vi "DB UI - Admin Equipment.vi"() -> ()   [LabVIEW 2013]
uses:
  Controls/Combo Box.ctl
  <vilib>/Utility/miscctls.llb/LVRowAndColumnUnsignedTypeDef.ctl
  <vilib>/Utility/miscctls.llb/LVRowAndColumnTypeDef.ctl
  <vilib>/Utility/miscctls.llb/LVPointTypeDef.ctl
  Controls/DB - [Admin].[Equipment] v20140922_1553.ctl
  Controls/Global SRTRS.vi
  <vilib>/addons/database/Connection.llb/DB Tools Open Connec (String).vi
  <vilib>/addons/database/Connection.llb/Conn Execute.vi
  <vilib>/addons/database/Recordset.llb/Rec Destroy - Connection.vi
  <vilib>/addons/database/Recordset.llb/Rec Fetch Recordset Data (R).vi
  <vilib>/addons/database/_DB Variant To Data/Database Variant To Data.xnode
  <vilib>/addons/database/NI_Database_API.lvlib
panel:
  in  "Search Equipment ID":T1
  in  "Tab Control":enum32{"Debug"}(tab)
  out "MHandler":errorcluster
  in  "Stop Button":bool
  out "Statemachine":errorcluster
  in  "# of Columns":i32=8
  out "Primary Keys":string[](array[string])=["OrderNo"]
  out "Foreign Keys":string[](array[string])=["OrderNo"]
  in  "Next Button":bool
  in  "Previous Button":bool
  out "1st Primary KEY":string
  in  "Last Button":bool
  in  "First Button":bool
  out "datetime string":string
  out "Changed":bool
  out "SQL Query":string
  in  "Include Inactive":bool=TRUE
  out "Extra Event From \"Select Foreign Key\"":bool
  out "IDENTITY COLUMN":string
  out "Close":errorcluster
  out "New Record in UI not in DB":bool
  out "Property Node":errorcluster
  out "DB":errorcluster
  in  "DB.Schema.Table":string="SRTRS.Admin.Equipment"
  in  "[PlantId]":string="4070"
  in  "DB.Schema.Table 2":string="SRTRS.Config.EquipmentType"
  in  "DB.Schema.Table 3":string="SRTRS.Config.System"
  out "Col Hdrs[] DB Data Type":string[](array[string])
  in  "# of Rows":u32=8
  out "Col Hdrs[] DB Precision":string[](array[string])
  out "All Mandatory Fields Filled":bool
  in  "------------------------------------        User Details Header EVENTS     ------------------------------------":string caption="------------------------------------        Setup Tab     ------------------------------------"
  in  "------------------------------------------        Unused EVENTS     ----------------------------------------":string caption="------------------------------------        Setup Tab     ------------------------------------"
  out "Connection Information":T2={"Connection "="SQL Server 32bit HPEnvy", "Username"="admin", "Password"="admin123"}
  out "MCListBox":u32
  out "NewVal":i32
  out "User Details":u32
  out "Controls (Caption) that are blank (Unicode)":string[](array[string])
  in  "Save Enabled depends on \nFilled Mandatory Fields":bool
  in  "CellBG New Cells":u32(colorbox)=16777225
  in  "CellBG Unused Cells":u32(colorbox)=16777238
  in  "CellBG ColHdrs":u32(colorbox)=11776947
  in  "Ascending":bool
  in  "List [CaptionOnly]":string caption="List"
  in  "Cal. History":bool caption="Setup Save"
  in  "Search System ID":T1
  in  "Save":bool caption="Setup Save"
  in  "New":bool caption="Setup Save"
  in  "Equipment Details Cluster":T3={"Equipment ID"="", "Equipment Name"="", "Plant ID"="", "Equipment Type"="", "System"="", "Manufacturer"="", "Model Number"="", "Serial Number"="", "Last Calibration"=timestamp(0 s since 1904-01-01), "Next Calibration"=timestamp(0 s since 1904-01-01), "Calibration Period"="", "Notice Period"="", "Registration Date"=timestamp(0 s since 1904-01-01), "Remarks"="", "Out For Calibration"=FALSE, "Required Calibration"=TRUE, "Inactive"=FALSE, "Equipment Type Name"="", "System Name"="", "Days1 [CaptionOnly]"="", "Days2 [CaptionOnly]"=""} caption="Record" {"Registration Date" format="%<%Y/%m/%d>T"; "Last Calibration" format="%<%Y/%m/%d>T"; "Next Calibration" format="%<%Y/%m/%d>T"}
  in  "Current Record":i32 caption="No."
  out "Record Count":i32
  in  "Multicolumn Listbox":i32(listbox)=3
  # "/"
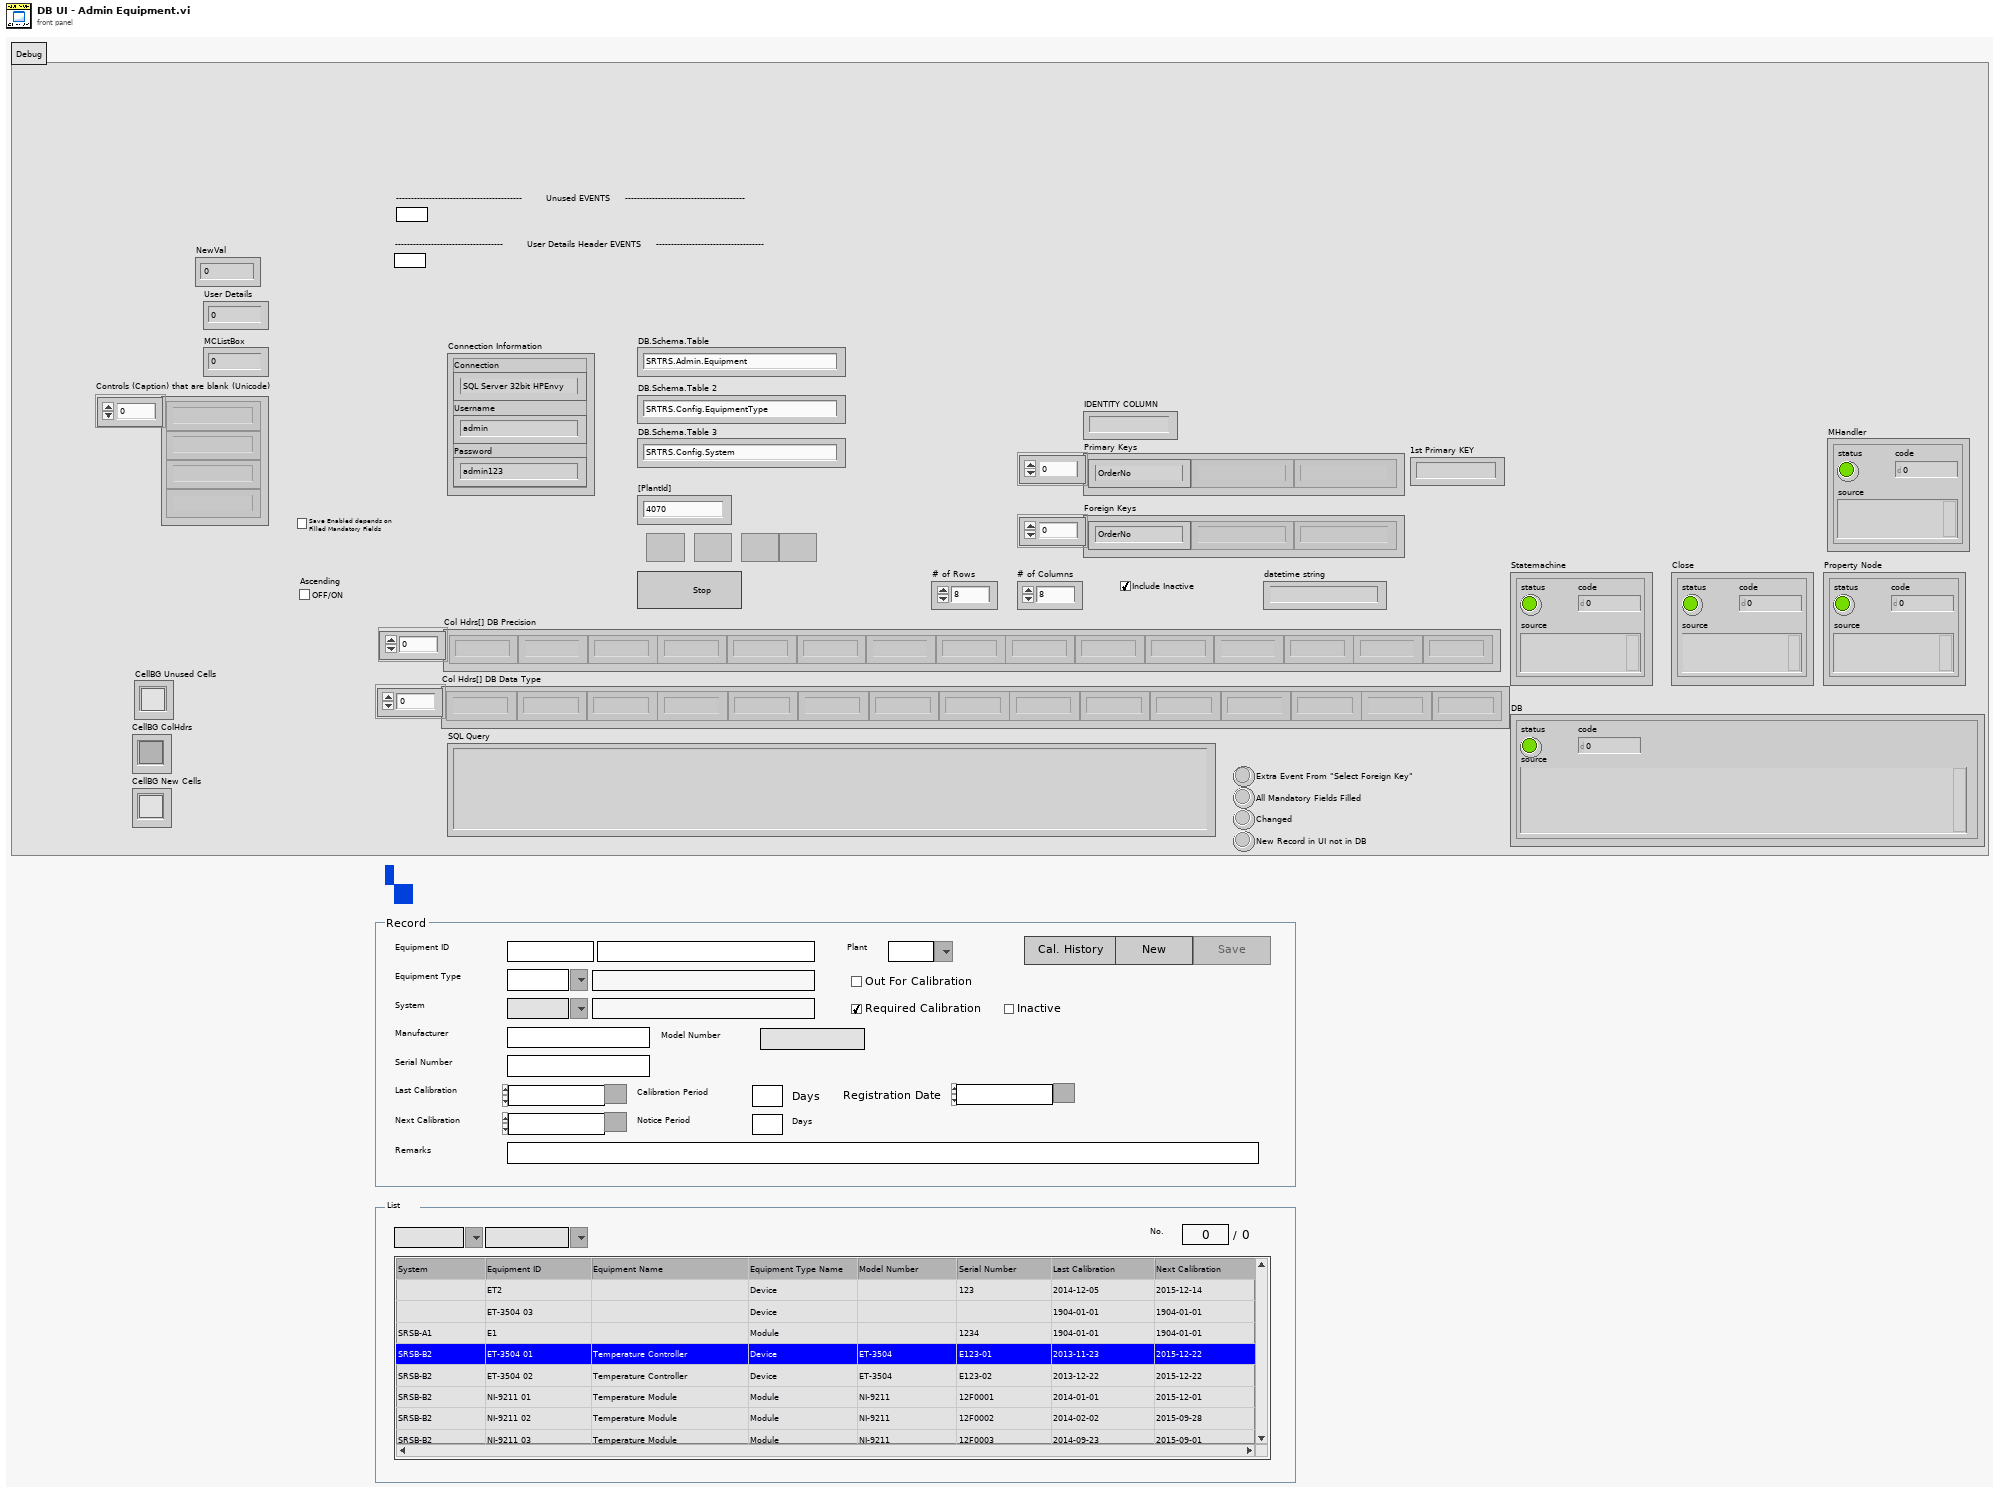
[diagram p1: front panel]
types:
  T1 = typedef "Combo Box.ctl" = string
  T2 = cluster{"Connection ":string, "Username":string, "Password":string}
  T3 = cluster{"Equipment ID":string, "Equipment Name":string, "Plant ID":T1, "Equipment Type":T1, "System":T1, "Manufacturer":string, "Model Number":string, "Serial Number":string, "Last Calibration":timestamp, "Next Calibration":timestamp, "Calibration Period":string, "Notice Period":string, "Registration Date":timestamp, "Remarks":string, "Out For Calibration":bool, "Required Calibration":bool, "Inactive":bool, "Equipment Type Name":string, "System Name":string, "Days1 [CaptionOnly]":string, "Days2 [CaptionOnly]":string}
  T4 = typedef "LVPointTypeDef.ctl" = cluster{"Horizontal":i16, "Vertical":i16}
  T5 = typedef "LVRowAndColumnUnsignedTypeDef.ctl" = cluster{"Row":u32, "Column":u32}
  T6 = enum8{"Enabled", "Disabled", "Disabled and Grayed Out"}
  T7 = typedef "DB - [Admin].[Equipment] v20140922_1553.ctl" = enum16{"a.[PlantId]", "a.[EquipmentId]", "a.[Description]", "a.[EquipmentTypeId]", "c.[ShortDescription]", "a.[SystemId]", "s.[Description]", "a.[Manufacturer]", "a.[Model]", "a.[SerialNo]", "a.[RegistrationDate]", "a.[IsCalibRequired]", "a.[IsCalibOut]", "a.[CalibrationPeriod]", "a.[NoticePeriod]", "a.[LastCalibDate]", "a.[NextCalibDate]", "a.[Remarks]", "a.[Inactive]"}
  T8 = typedef "LVRowAndColumnTypeDef.ctl" = cluster{"Row":i32, "Column":i32}
  T9 = typedef "Connection Information Cluster.ctl" = cluster{"Connection ":string, "Username":string, "Password":string}
  T10 = typedef "NI_Database_API.lvlib/Conn ObjectReference.ctl" = refnum<k1>
  T11 = typedef "DB - DB.Schema.Table.ctl" = cluster{"DB":string, "Schema":string, "Table":string}
  T12 = typedef "NI_Database_API.lvlib/Rec ObjectReference.ctl" = refnum<k1>
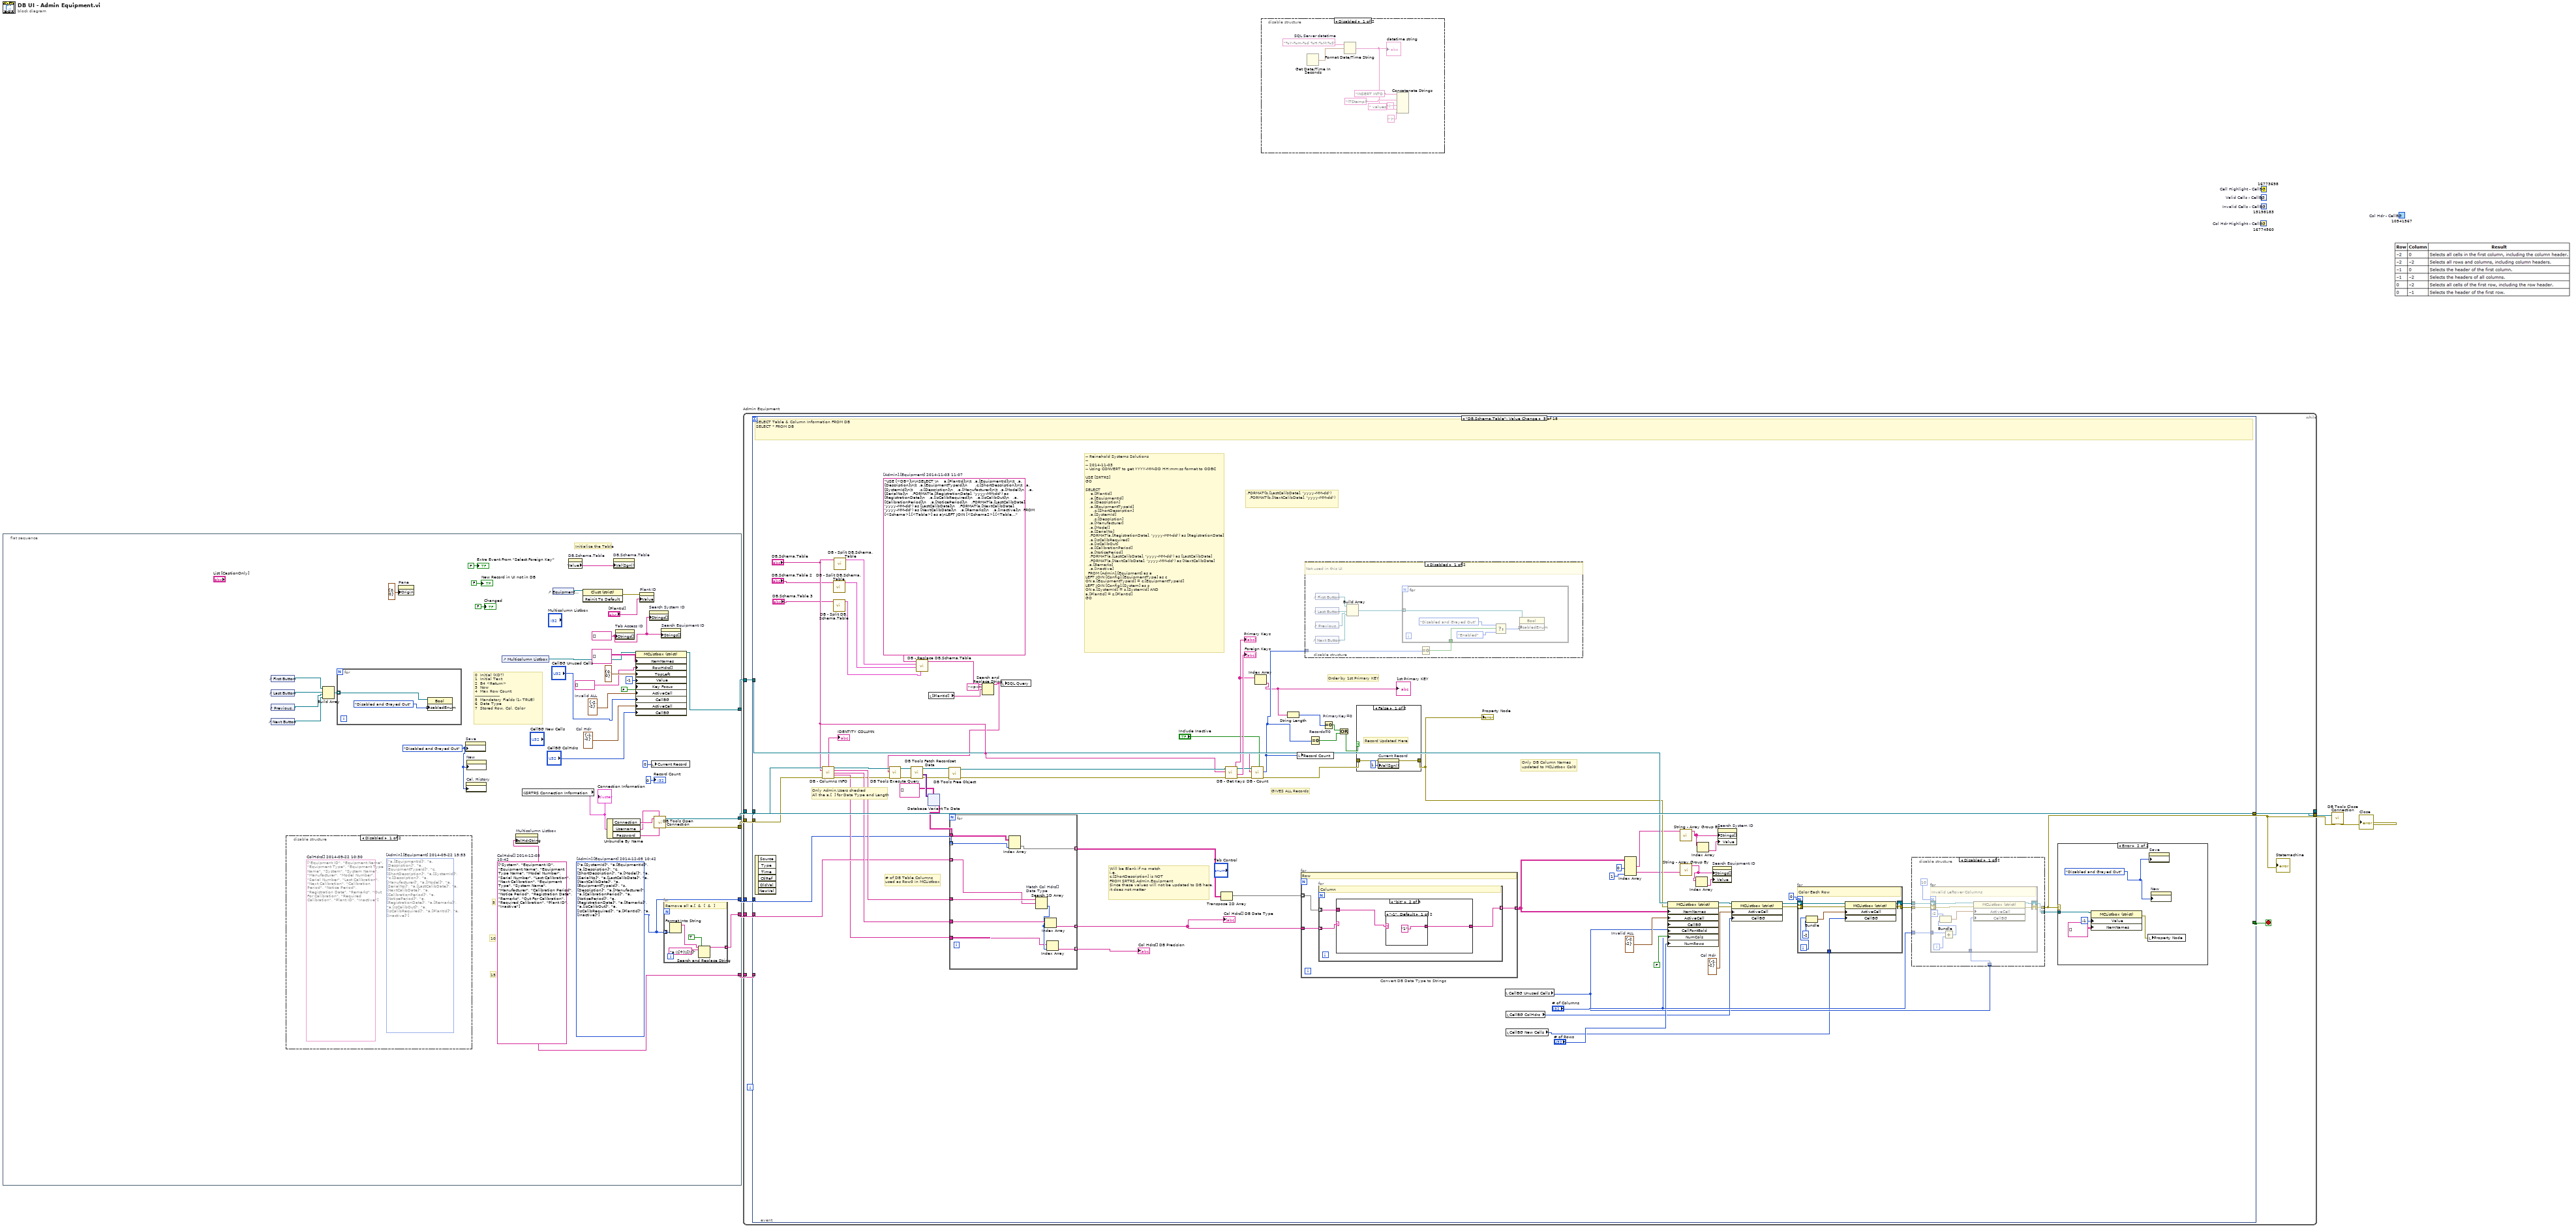
[diagram p0: block diagram]
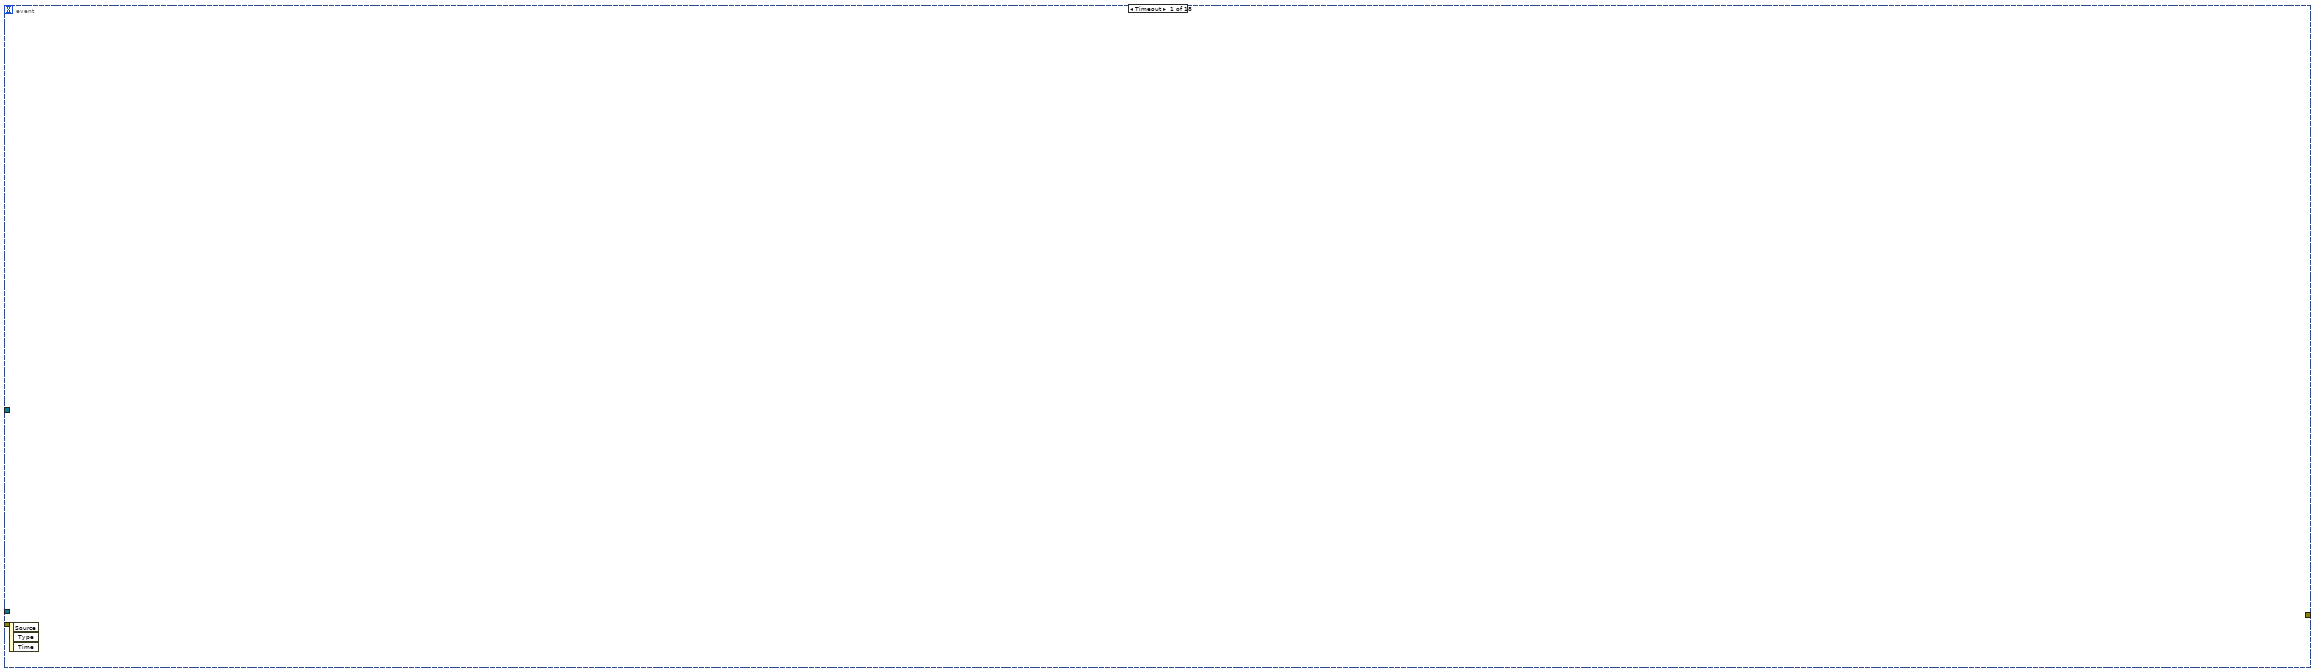
[diagram p4: hidden frame]
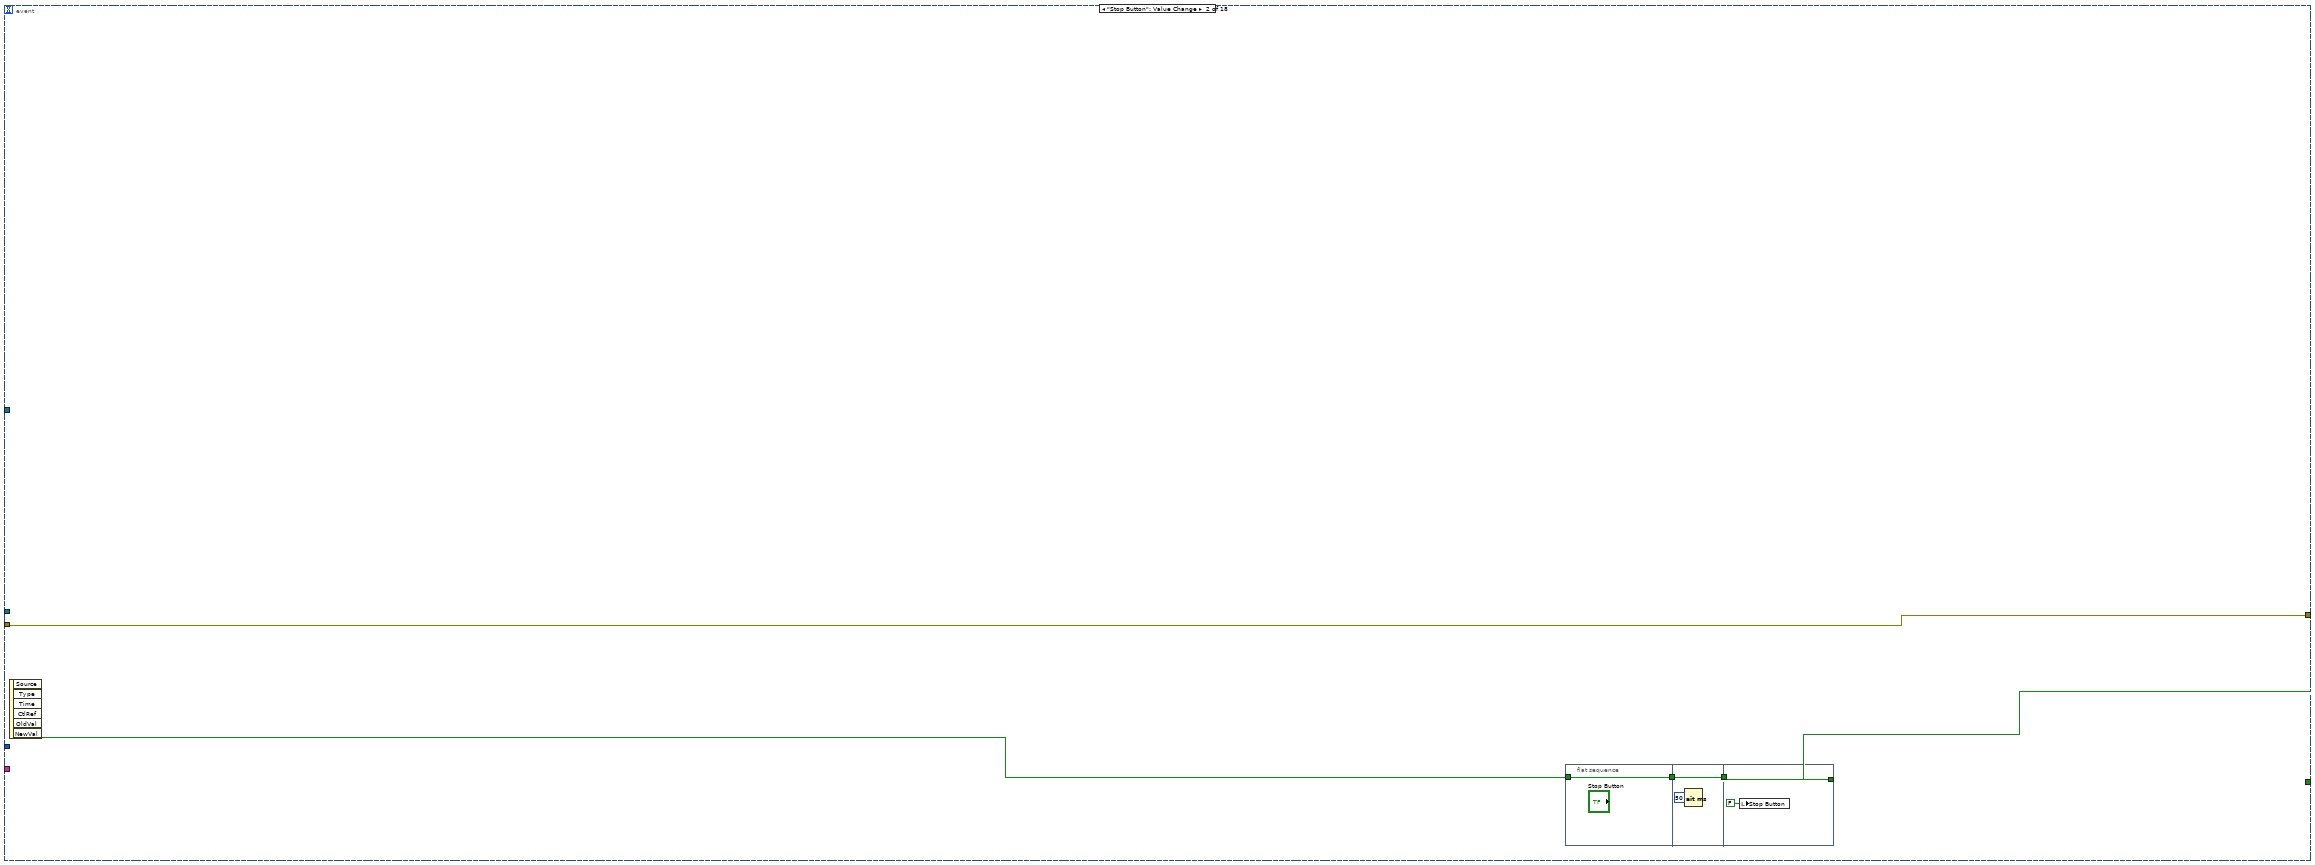
[diagram p5: hidden frame]
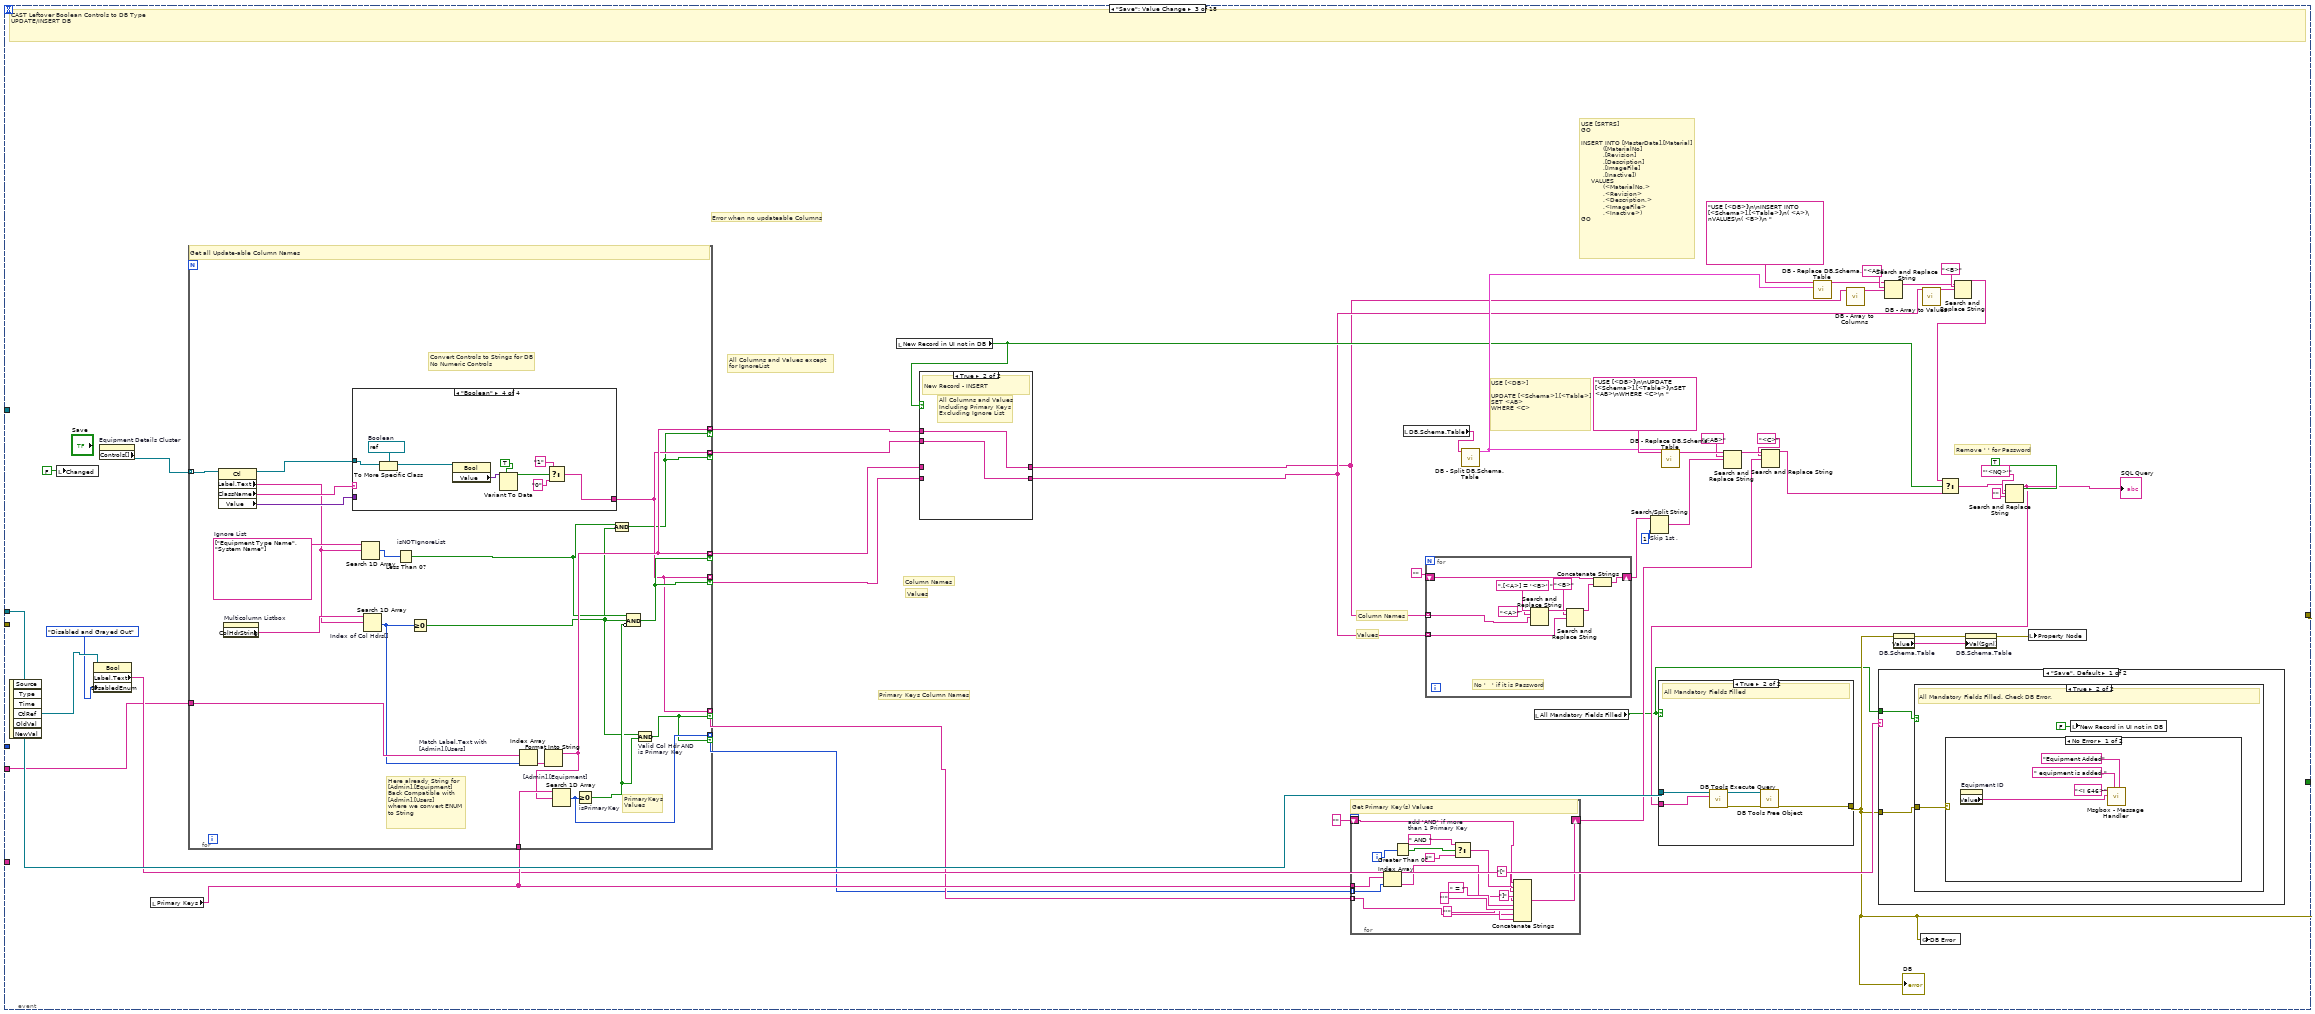
[diagram p6: hidden frame]
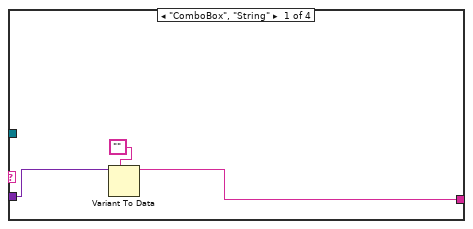
[diagram p8: hidden frame]
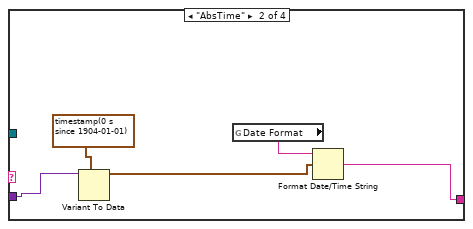
[diagram p9: hidden frame]
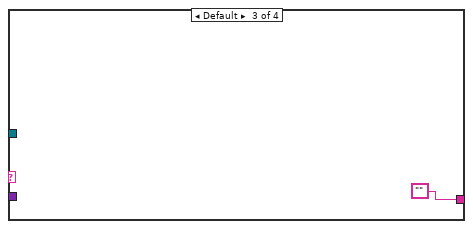
[diagram p10: hidden frame]
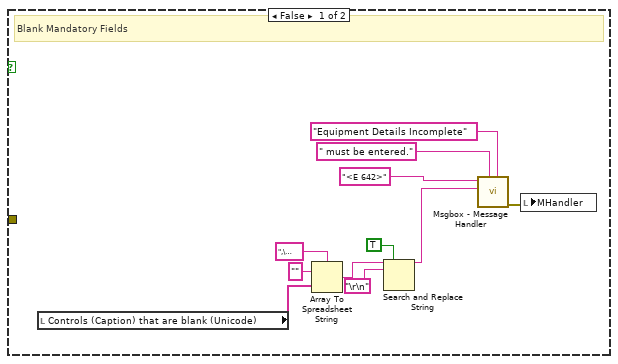
[diagram p12: hidden frame]
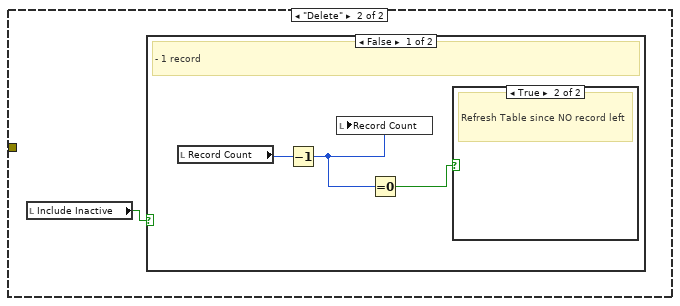
[diagram p14: hidden frame]
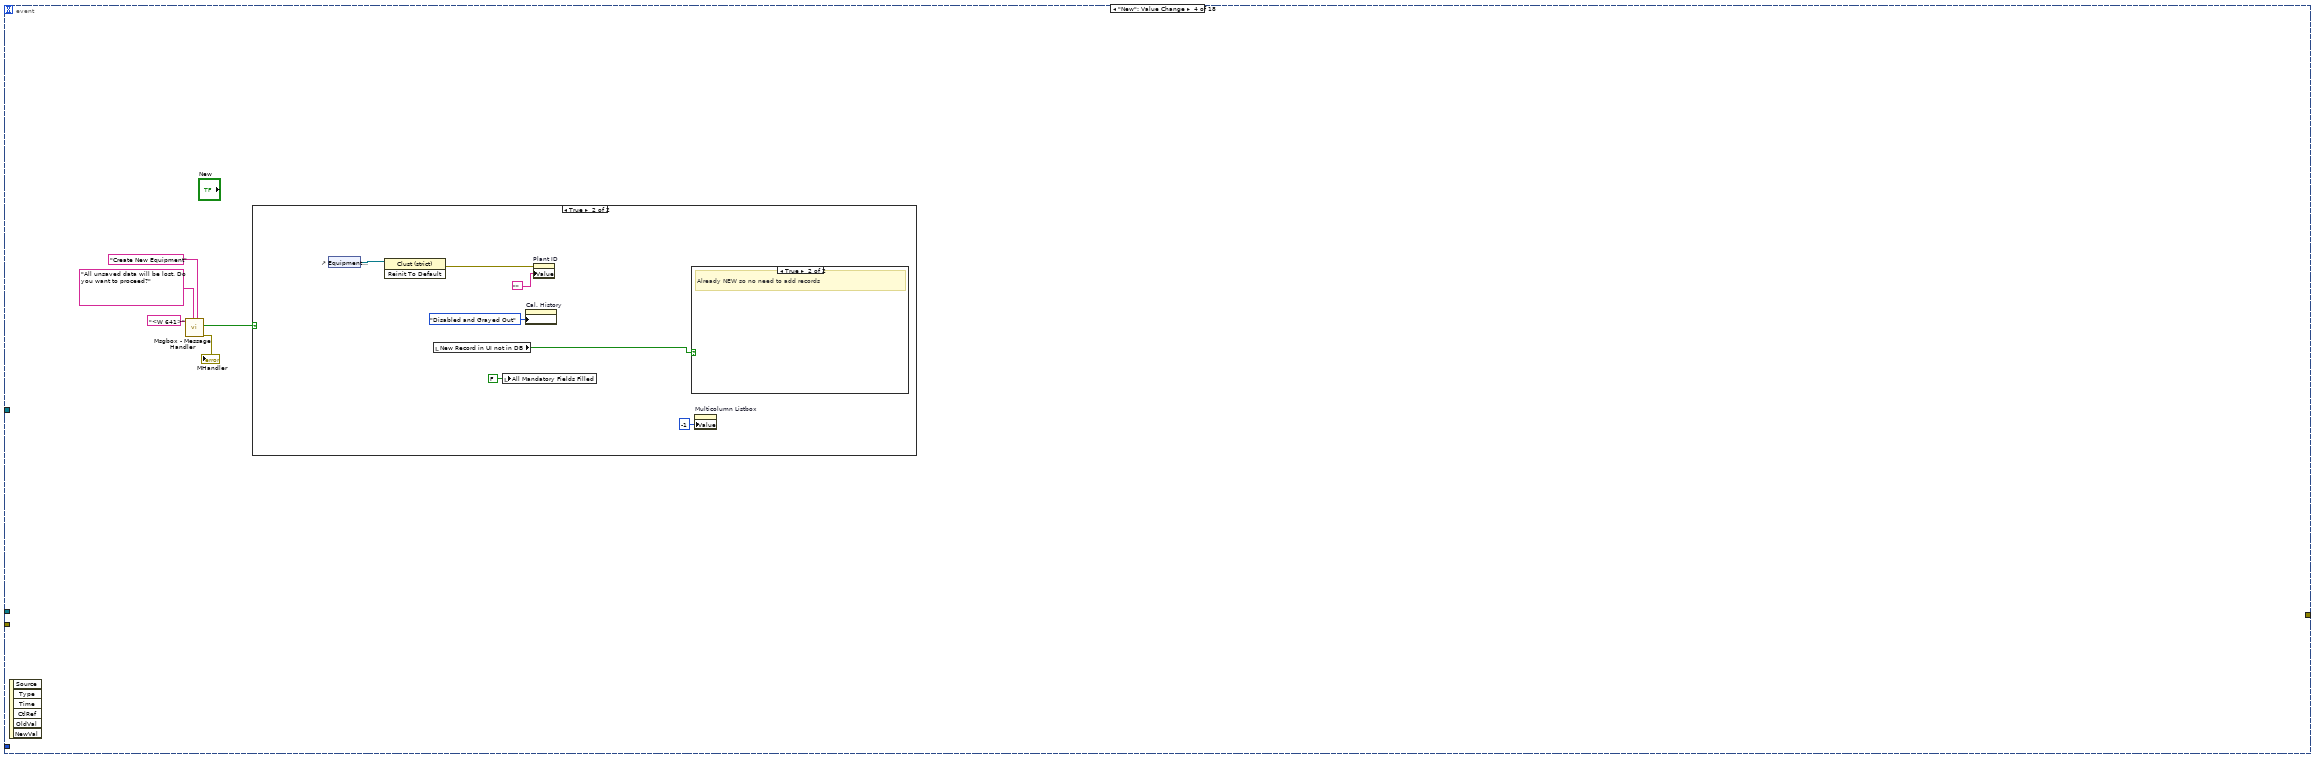
[diagram p17: hidden frame]
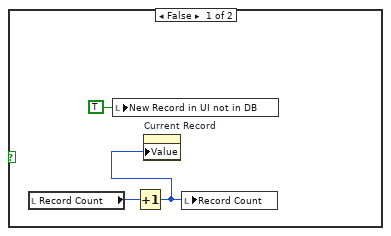
[diagram p19: hidden frame]
diagram:
  (unwired) u32 10541567  # Col Hdr - CellBG
  (unwired) u32 16777226  # Valid Cells - CellBG
  (unwired) u32 15198183  # Invalid Cells - CellBG
  (unwired) u32 16774560  # Col Hdr Highlight - CellBG
  (unwired) u32 16773698  # Cell Highlight - CellBG
  n1 = flat-sequence {
    tunnel: [w43] -> w9
    tunnel: [w23] -> w6
    tunnel: [w41] -> w5
    tunnel: [w16] -> w3
    tunnel: [w19] -> w2
    tunnel: [w15] -> w1
    frame #0 {
      w15 = T7[] [enum."a.[SystemId]", enum."a.[EquipmentId]", enum."a.[Description]", enum."c.[ShortDescription]", enum."a.[Model]", enum."a.[SerialNo]", enum."a.[LastCalibDate]", enum."a.[NextCalibDate]", enum."a.[EquipmentTypeId]", enum."s.[Description]", enum."a.[Manufacturer]", enum."a.[CalibrationPeriod]", enum."a.[NoticePeriod]", enum."a.[RegistrationDate]", enum."a.[Remarks]", enum."a.[IsCalibOut]", enum."a.[IsCalibRequired]", enum."a.[PlantId]", enum."a.[Inactive]"] items=["a.[PlantId]", "a.[EquipmentId]", "a.[Description]", "a.[EquipmentTypeId]", "c.[ShortDescription]", "a.[SystemId]", "s.[Description]", "a.[Manufacturer]", "a.[Model]", "a.[SerialNo]", "a.[RegistrationDate]", "a.[IsCalibRequired]", "a.[IsCalibOut]", "a.[CalibrationPeriod]", "a.[NoticePeriod]", "a.[LastCalibDate]", "a.[NextCalibDate]", "a.[Remarks]", "a.[Inactive]"]  # [Admin].[Equipment] 2014-12-05 10:42
      w10 = string[] [] ("Strings []")
      w19 = string[] ["System", "Equipment ID", "Equipment Name", "Equipment Type Name", "Model Number", "Serial Number", "Last Calibration", "Next Calibration", "Equipment Type", "System Name", "Manufacturer", "Calibration Period", "Notice Period", "Registration Date", "Remarks", "Out For Calibration", "Required Calibration", "Plant ID", "Inactive"]  # ColHdrs[] 2014-12-05 10:42
      w24 = T8 {"Row"=-1, "Column"=-2}  # Col Hdr
      w25 = T8 {"Row"=-2, "Column"=-2}  # Invalid ALL
      w13 = T6."Disabled and Grayed Out" ("Disabled")
      # "15"
      # "10"
      # "5"
      # "Initialize the Table"
      # "0  Initial (KD?)\n1  Initial Text\n2  B4 <Return>\n3  Now\n4  Max Row Count\n-------------------\n5  Mandatory Fields (1- TRUE)\n6  Data Type\n7  Stored Row, Col, Color"
      n2 = control-ref of="First Button"() -> (w37:refnum<vi>)
      n3 = control-ref of="Last Button"() -> (w36:refnum<vi>)
      n4 = control-ref of="Previous Button"() -> (w35:refnum<vi>)
      n5 = control-ref of="Next Button"() -> (w34:refnum<vi>)
      n6 = disable-structure shown="Disabled" {
        frame Disabled {
          (unwired) T7[] [enum."a.[EquipmentId]", enum."a.[Description]", enum."a.[EquipmentTypeId]", enum."c.[ShortDescription]", enum."a.[SystemId]", enum."s.[Description]", enum."a.[Manufacturer]", enum."a.[Model]", enum."a.[SerialNo]", enum."a.[LastCalibDate]", enum."a.[NextCalibDate]", enum."a.[CalibrationPeriod]", enum."a.[NoticePeriod]", enum."a.[RegistrationDate]", enum."a.[Remarks]", enum."a.[IsCalibOut]", enum."a.[IsCalibRequired]", enum."a.[PlantId]", enum."a.[Inactive]"] items=["a.[PlantId]", "a.[EquipmentId]", "a.[Description]", "a.[EquipmentTypeId]", "c.[ShortDescription]", "a.[SystemId]", "s.[Description]", "a.[Manufacturer]", "a.[Model]", "a.[SerialNo]", "a.[RegistrationDate]", "a.[IsCalibRequired]", "a.[IsCalibOut]", "a.[CalibrationPeriod]", "a.[NoticePeriod]", "a.[LastCalibDate]", "a.[NextCalibDate]", "a.[Remarks]", "a.[Inactive]"]  # [Admin].[Equipment] 2014-09-22 15:53
          (unwired) string[] ["Equipment ID", "Equipment Name", "Equipment Type", "Equipment Type Name", "System", "System Name", "Manufacturer", "Model Number", "Serial Number", "Last Calibration", "Next Calibration", "Calibration Period", "Notice Period", "Registration Date", "Remarks", "Out For Calibration", "Required Calibration", "Plant ID", "Inactive"]  # ColHdrs[] 2014-09-22 10:30
        }
        frame Enabled {
        }
      }
      n7 = Build Array(w37, w36, w35, w34) -> (w38:refnum<vi>[])
      n8 = for {
        tunnel: w38 -> [w53] mode=indexing
        n9 = property class="Bool"(reference=w53, "DisabledEnum"=T6."Disabled and Grayed Out" ("Disabled")) -> ()  [unwired: 1 in, 2 out]
      }
      n10 = property on="Pane" class="Pane"("Origin"=T4 {"Horizontal"=0, "Vertical"=0}) -> ()  [unwired: 2 in, 2 out]
      n11 = property on="Save" class="Bool"("DisabledEnum"=w13) -> ()  [unwired: 2 in, 2 out]
      n12 = property on="Cal. History" class="Bool"("DisabledEnum"=w13) -> ()  [unwired: 2 in, 2 out]
      n13 = property on="New" class="Bool"("DisabledEnum"=w13) -> ()  [unwired: 2 in, 2 out]
      n14 = control-ref of="Multicolumn Listbox"() -> (w22:refnum<vi>)
      n15 = property on="Multicolumn Listbox" class="MCListbox (strict)"("ColHdrString"=w19) -> ()  [unwired: 2 in, 2 out]
      n16 = global read "Global SRTRS.vi" "SRTRS Connection Information"() -> (w14:T9)
      "Connection Information" <- w14
      n17 = control-ref of="Equipment Details Cluster"() -> (w21:refnum<vi>)
      n18 = property on="DB.Schema.Table" class="Str"() -> ("Value"=w31:string)  [unwired: 2 in, 2 out]
      n19 = invoke class="Clust (strict)" method="Reinit To Default"(reference=w21) -> (error out=w20:errorcluster)  [unwired: 2 in, 2 out]
      n20 = Unbundle By Name(w14) -> ("Connection"=w46:string, "Username"=w45:string, "Password"=w44:string)
      n21 = property on="DB.Schema.Table" class="Str"("Val(Sgnl)"=w31) -> ()  [unwired: 2 in, 2 out]
      n22 = property on="Tab Access ID" class="CmbBox (strict)"("Strings[]"=w10) -> ()  [unwired: 2 in, 2 out]
      n23 = property on="Property Node" class="MCListbox (strict)"(reference=w22, "ItemNames"=string[][] [] ("Item Names"), "RowHdrs[]"=string[] [] ("Item Names"), "TopLeft"=T5 {"Row"=0, "Column"=0} ("Top Left Visible Cell"), "Value"=-1, "Key Focus"=FALSE, "ActiveCell"=w25, "CellBG"="CellBG Unused Cells", "ActiveCell"=w24, "CellBG"="CellBG ColHdrs") -> (reference out=w23:refnum<vi>)  [unwired: 1 in, 1 out]
      n24 = property on="Plant ID" class="CmbBox (strict)"(error in=w20, "Value"="[PlantId]") -> ()  [unwired: 1 in, 2 out]
      n25 = property on="Search System ID" class="CmbBox (strict)"("Strings[]"=w10) -> ()  [unwired: 2 in, 2 out]
      n26 = local write "Current Record"(0 ("Current Record")) -> ()
      n27 = call-poly <vilib>:"DB Tools Open Connection.vi"("password"=w44, "userID"=w45, "connection information"=w46) -> ("error out"=w41:errorcluster, "connection reference"=w43:T10)  [unwired: 5 in]
      n28 = property on="Search Equipment ID" class="CmbBox (strict)"("Strings[]"=w10) -> ()  [unwired: 2 in, 2 out]
      n29 = for {
        tunnel: w15 -> [w51] mode=indexing
        tunnel: [w47] -> w16 mode=indexing
        # "Remove all a.[  &  [  &  ]"
        n30 = Format Into String(w51) -> (resulting string=w48:string)  [unwired: 3 in, 1 out]
        n31 = Search and Replace String(replace all?=TRUE ("replace all? (F)"), input string=w48, search string="a.\\[+|\\[|\\]") -> (result string=w47:string)  [unwired: 5 in, 3 out]
      }
      "Extra Event From \"Select Foreign Key\"" <- FALSE ("Extra Event From \"Select Foreign Key Value Changed\"")
      "Record Count" <- 0 ("Record Count")
      "New Record in UI not in DB" <- FALSE ("New Record in UI not in DB")
      "Changed" <- FALSE ("Changed")
    }
  }
  n32 = while "Admin Equipment" {
    tunnel: w9 -> [w58]
    tunnel: [w58] -> w8
    tunnel: [w57] -> w7
    tunnel: w5 -> [w60]
    tunnel: w6 -> [w59]
    tunnel: w3 -> [w56]
    tunnel: w2 -> [w55]
    tunnel: w1 -> [w54]
    stop <- w61 stop-if-true
    n33 = event shown="[4] \"DB.Schema.Table\": Value Change" {
      selector: _ -> [_ _ _ _ _ _ _ _ _ _ _ _ _ _ _ _ _ _]
      dyn-events: _ -> [_ _ _ _ _ _ _ _ _ _ _ _ _ _ _ _ _ _]
      timeout: _ -> [_ _ _ _ _ _ _ _ _ _ _ _ _ _ _ _ _ _]
      tunnel: [_ w64 _ _ _ _ _ _ _ _ _ _ _ _ _ _ _ _] -> w61
      tunnel: w58 -> [_ _ w120 _ w293 _ _ _ _ _ _ w564 w630 _ _ _ _ w881]
      tunnel: [_ w66 w73 _ w280 _ _ _ w467 _ _ w545 _ _ _ _ _ _] -> w57
      tunnel: w60 -> [_ w66 _ _ w292 _ _ _ w468 _ _ _ _ _ _ _ _ w880]
      tunnel: w59 -> [_ _ _ _ w301 _ w446 _ w466 _ _ _ _ w720 _ w779 _ _]
      tunnel: w56 -> [_ _ w91 _ w272 _ _ _ _ _ _ w553 w650 _ _ _ _ _]
      tunnel: w55 -> [_ _ _ _ _ _ _ _ _ _ _ w556 w653 _ _ _ _ _]
      tunnel: w54 -> [_ _ _ _ w249 _ _ _ _ _ _ _ _ _ _ _ _ _]
      event Timeout {
        n34 = event-data() -> ()  [unwired: 1 in, 3 out]
      }
      event "Stop Button": Value Change {
        n35 = event-data() -> ("NewVal"=w65:bool)  [unwired: 1 in, 5 out]
        n36 = flat-sequence {
          tunnel: w65 -> [w67]
          tunnel: [w67] -> w62
          tunnel: [w68] -> w63
          tunnel: w62 -> [w68]
          tunnel: [w70] -> w64
          tunnel: w63 -> [w70]
          frame #0 {
          }
          frame #1 {
            n37 = Wait (ms)(milliseconds to wait=u32 50) -> ()  [unwired: 1 out]
          }
          frame #2 {
            n38 = local write "Stop Button"(FALSE ("Stop Button")) -> ()
          }
        }
      }
      event "Save": Value Change {
        # "All Columns and Values except\nfor IgnoreList"
        # "Primary Keys Column Names"
        # "Values"
        # "Column Names"
        # "Remove ' ' for Password"
        # "Values"
        # "Column Names"
        # "Error when no updateable Columns"
        # "USE [SRTRS]\nGO\n\nINSERT INTO [MasterData].[Material]\n           ([MaterialNo]\n           ,[Revision]\n           ,[Description]\n           ,[ImageFile]\n           ,[Inactive])\n     VALUES\n           (<MaterialNo,>\n           ,<Revision>\n           ,<Description,>\n           ,<ImageFile>\n           ,<Inactive>)\nGO"
        # "USE [<DB>]\n\nUPDATE [<Schema>].[<Table>]\nSET <AB>\nWHERE <C>"
        # "CAST Leftover Boolean Controls to DB Type\nUPDATE/INSERT DB"
        n39 = event-data() -> ("CtlRef"=w107:refnum<vi>)  [unwired: 1 in, 5 out]
        n40 = local write "Changed"(FALSE ("Changed")) -> ()
        n41 = property class="Bool"(reference=w107, "DisabledEnum"=T6."Disabled and Grayed Out" ("Disabled")) -> ("Label.Text"=w93:string)  [unwired: 1 in, 2 out]
        n42 = property on="Equipment Details Cluster" class="Clust (strict)"() -> ("Controls[]"=w85:refnum<vi>[])  [unwired: 2 in, 2 out]
        n43 = local read "Primary Keys"() -> (w108:string[])
        n44 = for {
          tunnel: [w133] -> w84 mode=indexing if=w141
          tunnel: w108 -> [w140]
          tunnel: w85 -> [w146] mode=indexing
          tunnel: w91 -> [w144]
          tunnel: [w132] -> w83 mode=indexing if=w141
          tunnel: [w132] -> w90 mode=indexing if=w134
          tunnel: [w135] -> w89 mode=indexing if=w134
          tunnel: [w133] -> w87 mode=indexing if=w130
          tunnel: [w132] -> w86 mode=indexing if=w130
          w138 = string[] ["Equipment Type Name", "System Name"]  # Ignore List
          # "Convert Controls to Strings for DB\nNo Numeric Controls"
          # "PrimaryKeys\nValues"
          # "Here already String for\n[Admin].[Equipment]\nBack Compatible with\n[Admin].[Users]\nwhere we convert ENUM \nto String"
          # "Get all Update-able Column Names"
          n45 = property class="Ctl"(reference=w146) -> (reference out=w127:refnum<vi>, "Label.Text"=w126:string, "ClassName"=w143:string, "Value"=w142:variant)  [unwired: 1 in, 1 out]
          n46 = property on="Multicolumn Listbox" class="MCListbox (strict)"() -> ("ColHdrString"=w145:string[])  [unwired: 2 in, 2 out]
          n47 = case shown="\"Boolean\"" w143 {
            tunnel: w142 -> [w147 w154 _ _]
            tunnel: [w148 w151 "" w156] -> w132
            tunnel: w127 -> [_ _ _ w164]
            frame "ComboBox", "String" {
              n48 = Variant To Data(type="", Variant=w147) -> (data=w148:string)  [unwired: 1 in, 1 out]
            }
            frame "AbsTime" {
              n49 = Variant To Data(type=timestamp(0 s since 1904-01-01), Variant=w154) -> (data=w150:timestamp)  [unwired: 1 in, 1 out]
              n50 = global read "Global SRTRS.vi" "Date Format"() -> (w152:string)
              n51 = Format Date/Time String(time format string (%c)=w152, seconds (now)=w150) -> (date/time string=w151:string)  [unwired: 1 in]
            }
            frame Default {
            }
            frame "Boolean" {
              w163 = refnum<vi> refnum  # Boolean
              n52 = To More Specific Class(target class=w163, reference=w164) -> (specific class reference=w162:refnum<vi>)  [unwired: 1 in, 1 out]
              n53 = property class="Bool"(reference=w162) -> ("Value"=w157:variant)  [unwired: 1 in, 2 out]
              n54 = Variant To Data(type=TRUE, Variant=w157) -> (data=w160:bool)  [unwired: 1 in, 1 out]
              n55 = Select(t="1", s=w160, f="0") -> (s? t:f=w156:string)
            }
          }
          n56 = Search 1D Array(1D array=w138, element=w126) -> (index of element=w139:i32)  [unwired: 1 in]
          n57 = Search 1D Array "Index of Col Hdrs[]"(1D array=w145, element=w126) -> (index of element=w128:i32)  [unwired: 1 in]
          n58 = Less Than 0? "isNOTIgnoreList"(x=w139) -> (x < 0?=w131:bool)
          n59 = Greater Or Equal To 0?(x=w128) -> (x >= 0?=w129:bool)
          n60 = Index Array "Match Label.Text with [Admin].[Users]"(array=w144, index=w128) -> (element=w137:string)
          n61 = Format Into String "[Admin].[Equipment]"(w137) -> (resulting string=w133:string)  [unwired: 3 in, 1 out]
          n62 = Search 1D Array(1D array=w140, element=w133) -> (index of element=w135:i32)  [unwired: 1 in]
          n63 = Greater Or Equal To 0? "isPrimaryKey"(x=w135) -> (x >= 0?=w136:bool)
          n64 = Compound Arithmetic op=AND(w131, w129) -> (w130:bool)
          n65 = Compound Arithmetic op=AND(w131, w129, invert w136) -> (w141:bool)
          n66 = Compound Arithmetic op=AND "Valid Col Hdr AND\nis Primary Key"(w129, w136) -> (w134:bool)
        }
        n67 = local read "New Record in UI not in DB"() -> (w88:bool)
        n68 = case shown="True" w88 {
          tunnel: w87 -> [_ w168]
          tunnel: w86 -> [_ w167]
          tunnel: w84 -> [w166 _]
          tunnel: w83 -> [w165 _]
          tunnel: [w166 w168] -> w74
          tunnel: [w165 w167] -> w82
          frame False {
            # "All Columns  and Values\nexcept for\nPrimary Keys Columns\nAND\nIgnore List"
            # "Existing Record - UPDATE"
          }
          frame True {
            # "All Columns and Values\nIncluding Primary Keys\nExcluding Ignore List"
            # "New Record - INSERT"
          }
        }
        n69 = for {
          tunnel: w108 -> [w196]
          shift-right: [w203] -> w109
          shift-left: "" -> [w198]
          tunnel: w90 -> [w197] mode=indexing
          tunnel: w89 -> [w195] mode=indexing
          i -> [w204]
          w201 = " AND "  # add 'AND' if more  than 1 Primary Key
          # "Get Primary Key(s) Values"
          n70 = Index Array(array=w196, index=w195) -> (element=w194:string)
          n71 = Greater Than 0?(x=w204) -> (x > 0?=w202:bool)
          n72 = Select(t=w201, s=w202, f="") -> (s? t:f=w199:string)
          n73 = Concatenate Strings(w198, w199, "[" ("string"), w194, "]" ("string"), " = " ("string"), "'" ("string"), w197, "'" ("string")) -> (w203:string)
        }
        n74 = local read "DB.Schema.Table"() -> (w92:string)
        n75 = for {
          tunnel: w82 -> [w213] mode=indexing
          shift-right: [w210] -> w117
          shift-left: "" -> [w212]
          tunnel: w74 -> [w209] mode=indexing
          # "No '   ' if it is Password"
          n76 = Search and Replace String(input string=",[<A>] = '<B>' ", search string="<A>", replace string=w209) -> (result string=w214:string)  [unwired: 5 in, 3 out]
          n77 = Search and Replace String(input string=w214, search string="<B>", replace string=w213) -> (result string=w211:string)  [unwired: 5 in, 3 out]
          n78 = Concatenate Strings(w212, w211) -> (w210:string)
        }
        n79 = call "DB - Split DB.Schema.Table.vi"("DB.Schema.Table"=w92) -> ("DB.Schema.Table"=w95:T11)  [unwired: 10 in]
        n80 = local read "All Mandatory Fields Filled"() -> (w72:bool)
        n81 = Search/Split String "Skip 1st ,"(string=w117, offset (0)=1) -> (match + rest of string=w112:string)  [unwired: 1 in, 2 out]
        n82 = call "DB - Replace DB.Schema.Table.vi"("DB.Schema.Table"=w95, "string in"="USE [<DB>]\n\nUPDATE [<Schema>].[<Table>]\nSET <AB>\nWHERE <C>\n ") -> ("string out"=w114:string)  [unwired: 8 in, 1 out]
        n83 = Search and Replace String(input string=w114, search string="<AB>", replace string=w112) -> (result string=w111:string)  [unwired: 5 in, 3 out]
        n84 = Search and Replace String(input string=w111, search string="<C>", replace string=w109) -> (result string=w98:string)  [unwired: 5 in, 3 out]
        n85 = call "DB - Replace DB.Schema.Table.vi"("DB.Schema.Table"=w95, "string in"="USE [<DB>]\n\nINSERT INTO [<Schema>].[<Table>]\n( <A>)\nVALUES\n( <B>)\n ") -> ("string out"=w96:string)  [unwired: 8 in, 1 out]
        n86 = call "DB - Array to Columns.vi"("Array"=w74) -> ("[Columns]"=w102:string)  [unwired: 10 in]
        n87 = Search and Replace String(input string=w96, search string="<A>", replace string=w102) -> (result string=w99:string)  [unwired: 5 in, 3 out]
        n88 = call "DB - Array to Values.vi"("Array (0xFFFE autodetect)"=w82) -> ("<Values>"=w101:string)  [unwired: 10 in]
        n89 = Search and Replace String(input string=w99, search string="<B>", replace string=w101) -> (result string=w78:string)  [unwired: 5 in, 3 out]
        n90 = Select(t=w78, s=w88, f=w98) -> (s? t:f=w77:string)
        n91 = Search and Replace String(replace all?=TRUE ("replace all? (F)"), input string=w77, search string="'<NQ>'", replace string="" ("replace string (\"\")")) -> (result string=w76:string)  [unwired: 4 in, 3 out]
        "SQL Query" <- w76
        n92 = case shown="True" w72 {
          tunnel: w120 -> [_ w125]
          tunnel: [_ w124] -> w73
          tunnel: w76 -> [_ w123]
          frame False {
            # "Blank Mandatory Fields"
          }
          frame True {
            # "All Mandatory Fields Filled"
            n93 = call-poly <vilib>:"DB Tools Execute Query.vi"("SQL query"=w123, "connection reference"=w125) -> ("error out"=w121:errorcluster, "recordset reference"=w122:T12)  [unwired: 6 in]
            n94 = call-poly <vilib>:"DB Tools Free Object.vi"("error in (no error)"=w121, "recordset reference"=w122) -> ("error out"=w124:errorcluster)  [unwired: 8 in, 1 out]
          }
        }
        "DB" <- w73
        n95 = case shown="\"Save\", Default" w93 {
          tunnel: w73 -> [w170 _]
          tunnel: w72 -> [w169 _]
          frame "Save", Default {
            n96 = case shown="True" w169 {
              tunnel: w170 -> [_ w182]
              frame False {
                # "Blank Mandatory Fields"
                n97 = local read "Controls (Caption) that are blank (Unicode)"() -> (w171:string[])
                n98 = Array To Spreadsheet String(delimiter (Tab)=",\u0000", array=w171, 3:"" ("format string")) -> (spreadsheet string=w176:string)
                n99 = Search and Replace String(replace all?=TRUE ("replace all? (F)"), input string=w176, search string="\r\n") -> (result string=w179:string)  [unwired: 5 in, 3 out]
                n100 = call "Msgbox - Message Handler.vi"("Short Description (When DB Not Available)"="Equipment Details Incomplete", "Description (When DB Not Available)"=" must be entered.", "Pre-Description"=w179, "<.?....> Message Code"="<E 642>") -> ("MHandler Error"=w181:errorcluster)  [unwired: 5 in, 2 out]
                n101 = local write "MHandler"(w181) -> ()
              }
              frame True {
                # "All Mandatory Fields Filled. Check DB Error."
                n102 = case shown="No Error" w182 {
                  frame No Error {
                    n103 = property on="Equipment ID" class="Str"() -> ("Value"=w184:string)  [unwired: 2 in, 2 out]
                    n104 = call "Msgbox - Message Handler.vi"("Short Description (When DB Not Available)"="Equipment Added", "Description (When DB Not Available)"=" equipment is added.", "Pre-Description"=w184, "<.?....> Message Code"="<I 646>") -> ()  [unwired: 5 in, 3 out]
                  }
                  frame Error {
                  }
                }
                n105 = local write "New Record in UI not in DB"(FALSE ("New Record in UI not in DB")) -> ()
              }
            }
          }
          frame "Delete" {
            n106 = local read "Include Inactive"() -> (w188:bool)
            n107 = case shown="False" w188 {
              frame False {
                # "- 1 record"
                n108 = local read "Record Count"() -> (w191:i32)
                n109 = Decrement(x=w191) -> (x-1=w190:i32)
                n110 = local write "Record Count"(w190) -> ()
                n111 = Equal To 0?(x=w190) -> (x = 0?=w189:bool)
                n112 = case shown="True" w189 {
                  frame False {
                  }
                  frame True {
                    # "Refresh Table since NO record left"
                  }
                }
              }
              frame True {
                # "No Change"
              }
            }
          }
        }
        n113 = property on="DB.Schema.Table" class="Str"(error in=w73) -> (error out=w105:errorcluster, "Value"=w104:string)  [unwired: 1 in, 1 out]
        n114 = global write "Global SRTRS.vi" "DB Error"(w73) -> ()
        n115 = property on="DB.Schema.Table" class="Str"(error in=w105, "Val(Sgnl)"=w104) -> (error out=w94:errorcluster)  [unwired: 1 in, 1 out]
        n116 = local write "Property Node"(w94) -> ()
      }
      event "New": Value Change {
        n117 = event-data() -> ()  [unwired: 1 in, 6 out]
        n118 = call "Msgbox - Message Handler.vi"("Short Description (When DB Not Available)"="Create New Equipment", "Description (When DB Not Available)"="All unsaved data will be lost. Do you want to proceed?", "<.?....> Message Code"="<W 641>") -> ("MHandler Error"=→"MHandler":errorcluster, "OK Out"=w218:bool)  [unwired: 6 in, 1 out]
        n119 = case shown="True" w218 {
          frame False {
          }
          frame True {
            n120 = control-ref of="Equipment Details Cluster"() -> (w227:refnum<vi>)
            n121 = invoke class="Clust (strict)" method="Reinit To Default"(reference=w227) -> (error out=w225:errorcluster)  [unwired: 2 in, 2 out]
            n122 = local read "New Record in UI not in DB"() -> (w226:bool)
            n123 = local write "All Mandatory Fields Filled"(FALSE ("All Mandatory Fields Filled")) -> ()
            n124 = property on="Cal. History" class="Bool"("DisabledEnum"=T6."Disabled and Grayed Out" ("Disabled")) -> ()  [unwired: 2 in, 2 out]
            n125 = property on="Plant ID" class="CmbBox (strict)"(error in=w225, "Value"="") -> ()  [unwired: 1 in, 2 out]
            n126 = case shown="True" w226 {
              frame False {
                n127 = local read "Record Count"() -> (w231:i32)
                n128 = local write "New Record in UI not in DB"(TRUE ("New Record in UI not in DB")) -> ()
                n129 = Increment(x=w231) -> (x+1=w230:i32)
                n130 = property on="Current Record" class="DigNum (strict)"("Value"=w230) -> ()  [unwired: 2 in, 2 out]
                n131 = local write "Record Count"(w230) -> ()
              }
              frame True {
                # "Already NEW so no need to add records"
              }
            }
            n132 = property on="Multicolumn Listbox" class="MCListbox (strict)"("Value"=-1 ("Multicolumn Listbox")) -> ()  [unwired: 2 in, 2 out]
          }
        }
      }
      event "DB.Schema.Table": Value Change {
        w265 = "USE [<DB>]\n\nSELECT \n    a.[PlantId]\n\t  ,a.[EquipmentId]\n\t  ,a.[Description]\n\t  ,a.[EquipmentTypeId]\n      ,c.[ShortDescription]\n\t  ,a.[SystemId]\n\t     ,s.[Description]\n   ,a.[Manufacturer]\n\t  ,a.[Model]\n   ,a.[SerialNo]\n   ,FORMAT(a.[RegistrationDate], 'yyyy-MM-dd') as [RegistrationDate]\n   ,a.[IsCalibRequired]\n   ,a.[IsCalibOut]\n   ,a.[CalibrationPeriod]\n   ,a.[NoticePeriod]\n   ,FORMAT(a.[LastCalibDate], 'yyyy-MM-dd') as [LastCalibDate]\n   ,FORMAT(a.[NextCalibDate], 'yyyy-MM-dd') as [NextCalibDate]\n   ,a.[Remarks]\n   ,a.[Inactive]\n  FROM [<Schema>].[<Table>] as a\nLEFT JOIN [<Schema2>].[<Table2>] as c\nON a.[EquipmentTypeId] = c.[EquipmentTypeId]\nLEFT JOIN [<Schema3>].[<Table3>] as s\nON a.[SystemId] = s.[SystemId] AND\na.[PlantId] = s.[PlantId]\nWHERE a.[PlantId] = '<P>'\nORDER BY a.[SystemId], a.[EquipmentId]\n"  # [Admin].[Equipment] 2014-11-03 11:07
        w294 = T8 {"Row"=-1, "Column"=-2}  # Col Hdr
        w305 = T8 {"Row"=-2, "Column"=-2}  # Invalid ALL
        # ",FORMAT(b.[LastCalibDate], 'yyyy-MM-dd')\n  ,FORMAT(b.[NextCalibDate], 'yyyy-MM-dd')"
        # "-- Reinehold Systems Solutions\n-- \n-- 2014-11-03\n-- Using CONVERT to get YYYY-MM-DD HH:mm:ss format to ODBC\n\nUSE [SRTRS]\nGO\n\nSELECT \n    a.[PlantId]\n\t  ,a.[EquipmentId]\n\t  ,a.[Description]\n\t  ,a.[EquipmentTypeId]\n      ,c.[ShortDescription]\n\t  ,a.[SystemId]\n\t     ,s.[Description]\n   ,a.[Manufacturer]\n\t  ,a.[Model]\n   ,a.[SerialNo]\n   ,FORMAT(a.[RegistrationDate], 'yyyy-MM-dd') as [RegistrationDate]\n   ,a.[IsCalibRequired]\n   ,a.[IsCalibOut]\n   ,a.[CalibrationPeriod]\n   ,a.[NoticePeriod]\n   ,FORMAT(a.[LastCalibDate], 'yyyy-MM-dd') as [LastCalibDate]\n   ,FORMAT(a.[NextCalibDate], 'yyyy-MM-dd') as [NextCalibDate]\n  ,a.[Remarks]\n   ,a.[Inactive]\n  FROM [Admin].[Equipment] as a\nLEFT JOIN [Config].[EquipmentType] as c\nON a.[EquipmentTypeId] = c.[EquipmentTypeId]\nLEFT JOIN [Config].[System] as s\nON a.[SystemId] = s.[SystemId] AND\na.[PlantId] = s.[PlantId]\nGO"
        # "GIVES ALL Records"
        # "Will be Blank if no match\ni.e.\nc.[ShortDescription] is NOT \nFROM SRTRS.Admin.Equipment\nSince these values will not be updated to DB here, \nit does not matter"
        # "Only Admin.Users checked\nAll the a.[  ] for Data Type and Length"
        # "Only DB Column Names \nupdated to MCListbox Col0"
        # "Order by 1st Primary KEY"
        # "# of DB Table Columns\nused as Row0 in MCListbox"
        # "SELECT Table & Column Information FROM DB\nSELECT * FROM DB"
        n133 = event-data() -> ()  [unwired: 1 in, 6 out]
        n134 = call "DB - Columns INFO.vi"("Refnum in"=w293, "DB.dbo.Table"="DB.Schema.Table", "error in (no error)"=w292) -> ("IDENTITY COLUMN"=→"IDENTITY COLUMN":string, "Refnum out"=w263:T10, "COLUMN_NAME"=w274:string[], "DATA_TYPE"=w273:string[], "PRECISION"=w253:string[], "error out"=w257:errorcluster)  [unwired: 4 in, 3 out]
        n135 = call "DB - Split DB.Schema.Table.vi"("DB.Schema.Table"="DB.Schema.Table 2") -> ("DB.Schema.Table"=w251:T11)  [unwired: 10 in]
        n136 = call "DB - Split DB.Schema.Table.vi"("DB.Schema.Table"="DB.Schema.Table 3") -> ("DB.Schema.Table"=w250:T11)  [unwired: 10 in]
        n137 = call "DB - Split DB.Schema.Table.vi"("DB.Schema.Table"="DB.Schema.Table") -> ("DB.Schema.Table"=w258:T11)  [unwired: 10 in]
        n138 = call "DB - Replace DB.Schema.Table.vi"("DB.Schema.Table 3"=w250, "DB.Schema.Table 2"=w251, "DB.Schema.Table"=w258, "string in"=w265) -> ("string out"=w235:string)  [unwired: 6 in, 1 out]
        n139 = local read "[PlantId]"() -> (w232:string)
        n140 = Search and Replace String(input string=w235, search string="<P>", replace string=w232) -> (result string=w233:string)  [unwired: 5 in, 3 out]
        n141 = call-poly <vilib>:"DB Tools Execute Query.vi"("error in (no error)"=w257, "SQL query"=w233, "connection reference"=w263) -> ("error out"=w271:errorcluster, "recordset reference"=w270:T12)  [unwired: 5 in]
        n142 = call-poly <vilib>:"DB Tools Fetch Recordset Data.vi"("error in (no error)"=w271, "recordset reference"=w270) -> ("error out"=w266:errorcluster, "recordset data"=w269:variant[][], "recordset reference out"=w267:T12)  [unwired: 3 in]
        n143 = xnode "Database Variant To Data"("database variant"=w269, "type"=string[][] []) -> ("data"=w264:string[][])  [unwired: 1 in, 1 out]
        n144 = call-poly <vilib>:"DB Tools Free Object.vi"("error in (no error)"=w266, "recordset reference"=w267) -> ("error out"=w256:errorcluster, "connection reference"=w262:T10)  [unwired: 8 in]
        n145 = for {
          tunnel: w264 -> [w406]
          tunnel: w272 -> [w398] mode=indexing
          tunnel: [w405] -> w276 mode=indexing
          tunnel: w274 -> [w404]
          tunnel: w273 -> [w403]
          tunnel: [w402] -> w247 mode=indexing
          tunnel: w253 -> [w400]
          tunnel: [w399] -> w252 mode=indexing
          tunnel: w249 -> [w397] mode=indexing
          n146 = Index Array(array=w406, index (col)=w397) -> (element=w405:string[])  [unwired: 1 in]
          n147 = Search 1D Array "Match Col Hdrs[]\nData Type"(1D array=w404, element=w398) -> (index of element=w401:i32)  [unwired: 1 in]
          n148 = Index Array(array=w403, index=w401) -> (element=w402:string)
          n149 = Index Array(array=w400, index=w401) -> (element=w399:string)
        }
        "Col Hdrs[] DB Data Type" <- w247
        "Col Hdrs[] DB Precision" <- w252
        n150 = local write "SQL Query"(w233) -> ()
        n151 = Transpose 2D Array(2D array=w276) -> (transposed array=w248:string[][])
        n152 = call "DB - Get Keys.vi"("error in (no error)"=w256, "DB.Schema.Table"="DB.Schema.Table", "Refnum in"=w262) -> ("error out"=w298:errorcluster, "Foreign Keys"=→"Foreign Keys":string[], "Primary Key"=w290:string[], "Refnum out"=w299:T10)  [unwired: 5 in]
        "Primary Keys" <- w290
        n153 = call "DB - Count.vi"("Include Inactive"="Include Inactive", "error in (no error)"=w298, "DB.dbo.Table"="DB.Schema.Table", "Refnum in"=w299) -> ("error out"=w288:errorcluster, "COUNT"=w287:i32)  [unwired: 5 in, 1 out]
        n154 = Index Array(array=w290) -> (element=w286:string)  [unwired: 1 in]
        "1st Primary KEY" <- w286
        n155 = String Length(string=w286) -> (length=w285:i32)
        n156 = local write "Record Count"(w287) -> ()
        n157 = for "Convert DB Data Type to Strings" {
          tunnel: w248 -> [w327] mode=indexing
          tunnel: w247 -> [w326]
          tunnel: [w325] -> w246 mode=indexing
          # "Row"
          n158 = for {
            tunnel: w327 -> [w329] mode=indexing
            tunnel: w326 -> [w330] mode=indexing
            tunnel: [w328] -> w325 mode=indexing
            # "Column"
            n159 = case shown="\"bit\"" w330 {
              tunnel: w329 -> [w331 w333 w337]
              tunnel: [w331 w332 w336] -> w328
              frame "False", Default {
              }
              frame "bit" {
                n160 = case shown="\"-1\", Default" w333 {
                  selector: w333 -> [_ w335]
                  tunnel: ["1" w335] -> w332
                  frame "-1", Default {
                  }
                  frame "0" {
                  }
                }
              }
              frame "datetime", "datetime2" {
                # "SQL Server Default"
                n161 = Equal?(x=w337, y="1900-01-01") -> (x = y?=w339:bool)
                n162 = Select(t="", s=w339, f=w337) -> (s? t:f=w336:string)
              }
            }
          }
        }
        n163 = disable-structure shown="Disabled" {
          disable-tunnel: w287 -> [w341 _]
          frame Disabled {
            # "Not used in this UI"
            n164 = control-ref of="First Button"() -> (w347:refnum<vi>)
            n165 = control-ref of="Last Button"() -> (w346:refnum<vi>)
            n166 = control-ref of="Previous Button"() -> (w345:refnum<vi>)
            n167 = control-ref of="Next Button"() -> (w344:refnum<vi>)
            n168 = Build Array(w347, w346, w345, w344) -> (w343:refnum<vi>[])
            n169 = Equal To 0?(x=w341) -> (x = 0?=w342:bool)
            n170 = for {
              tunnel: w343 -> [w352] mode=indexing
              tunnel: w342 -> [w351]
              n171 = Select(t=T6."Disabled and Grayed Out" ("Disabled"), s=w351, f=T6."Enabled" ("Disabled")) -> (s? t:f=w348:T6)
              n172 = property class="Bool"(reference=w352, "DisabledEnum"=w348) -> ()  [unwired: 1 in, 2 out]
            }
          }
          frame Enabled {
          }
        }
        n173 = Equal To 0? "Records=0"(x=w287) -> (x = 0?=w283:bool)
        n174 = Equal To 0? "PrimaryKey=0"(x=w285) -> (x = 0?=w284:bool)
        n175 = Or(x=w284, y=w283) -> (x .or. y?=w282:bool)
        n176 = case shown="False" w282 {
          tunnel: w288 -> [w414 w417]
          tunnel: [w413 w417] -> w278
          frame False {
            # "Record Updated Here"
            n177 = property on="Current Record" class="DigNum (strict)"(error in=w414, "Val(Sgnl)"=1) -> (error out=w413:errorcluster)  [unwired: 1 in, 1 out]
          }
          frame True {
            # "No Primary KEY\nor No Records"
            n178 = local write "Current Record"(0 ("Current Record")) -> ()
          }
        }
        "Property Node" <- w278
        n179 = local read "CellBG Unused Cells"() -> (w244:u32)
        n180 = local read "CellBG ColHdrs"() -> (w245:u32)
        n181 = local read "CellBG New Cells"() -> (w243:u32)
        n182 = Index Array(array=w246, index (col) #1=0 ("disabled index (col)"), index (col) #2=1 ("disabled index (col)")) -> (element #1=w241:string[], element #2=w240:string[])  [unwired: 2 in]
        n183 = property on="Property Node" class="MCListbox (strict)"(reference=w301, error in=w278, "ItemNames"=w246, "ActiveCell"=w305, "CellBG"=w244, "CellFontBold"=FALSE ("Active Cell:Cell Font:Bold"), "NumCols"="# of Columns", "NumRows"="# of Rows") -> (reference out=w297:refnum<vi>, error out=w296:errorcluster)
        n184 = call "String - Array Group By.vi"("Array in"=w241) -> ("GROUP BY (Array in)"=w239:string[])  [unwired: 10 in]
        n185 = call "String - Array Group By.vi"("Array in"=w240) -> ("GROUP BY (Array in)"=w237:string[])  [unwired: 10 in]
        n186 = Index Array(array=w237) -> (element=w236:string)  [unwired: 1 in]
        n187 = Index Array(array=w239) -> (element=w238:string)  [unwired: 1 in]
        n188 = property on="Search Equipment ID" class="CmbBox (strict)"("Strings[]"=w237, "Value"=w236) -> ()  [unwired: 2 in, 2 out]
        n189 = property on="Search System ID" class="CmbBox (strict)"("Strings[]"=w239, "Value"=w238) -> ()  [unwired: 2 in, 2 out]
        n190 = property on="Property Node" class="MCListbox (strict)"(reference=w297, error in=w296, "ActiveCell"=w294, "CellBG"=w245) -> (reference out=w277:refnum<vi>, error out=w295:errorcluster)
        n191 = for {
          N: 0 -> [_]
          tunnel: w243 -> [w420]
          shift-right: [w424] -> w304
          shift-left: w295 -> [w425]
          shift-right: [w418] -> w303
          shift-left: w277 -> [w419]
          i -> [w423]
          # "Color Each Row"
          n192 = Bundle(w423, -2) -> (w421:cluster{i32, i32})  [unwired: 1 in]
          n193 = property on="Property Node" class="MCListbox (strict)"(reference=w419, error in=w425, "ActiveCell"=w421, "CellBG"=w420) -> (reference out=w418:refnum<vi>, error out=w424:errorcluster)
        }
        n194 = disable-structure shown="Disabled" {
          disable-tunnel: w304 -> [w312 w323]
          disable-tunnel: w303 -> [w310 w324]
          disable-tunnel: "# of Columns" -> [w309 _]
          disable-tunnel: [w308 w323] -> w280
          disable-tunnel: [w307 w324] -> w279
          disable-tunnel: w244 -> [w306 _]
          frame Disabled {
            n195 = for {
              N: 10 -> [_]
              tunnel: w306 -> [w318]
              tunnel: w309 -> [w316]
              shift-right: [w321] -> w308
              shift-left: w312 -> [w322]
              shift-right: [w313] -> w307
              shift-left: w310 -> [w314]
              i -> [w317]
              # "Invalid Leftover Columns"
              n196 = Add(x=w316, y=w317) -> (x+y=w315:i32)
              n197 = Bundle(-2, w315) -> (w320:cluster{i32, i32})  [unwired: 1 in]
              n198 = property on="Property Node" class="MCListbox (strict)"(reference=w314, error in=w322, "ActiveCell"=w320, "CellBG"=w318) -> (reference out=w313:refnum<vi>, error out=w321:errorcluster)
            }
          }
          frame Enabled {
          }
        }
        n199 = case shown="Error" w280 {
          tunnel: w279 -> [_ w412]
          frame No Error {
            n200 = property on="New" class="Bool"("DisabledEnum"=T6."Enabled" ("Disabled")) -> ()  [unwired: 2 in, 2 out]
          }
          frame Error {
            w409 = T6."Disabled and Grayed Out" ("Disabled")
            n201 = property on="Property Node" class="MCListbox (strict)"(reference=w412, "Value"=-1, "ItemNames"=string[][] [] ("Item Names")) -> (error out=w408:errorcluster)  [unwired: 1 in, 1 out]
            n202 = local write "Property Node"(w408) -> ()
            n203 = property on="Save" class="Bool"("DisabledEnum"=w409) -> ()  [unwired: 2 in, 2 out]
            n204 = property on="New" class="Bool"("DisabledEnum"=w409) -> ()  [unwired: 2 in, 2 out]
          }
        }
      }
      event "Multicolumn Listbox": Mouse Up {
        # "Mouse Up seems to work BEST for Sorting"
        n205 = event-data() -> ("CtlRef"=w430:refnum<vi>)  [unwired: 1 in, 7 out]
        n206 = control-ref of="Ascending"() -> (w431:refnum<vi>)
        n207 = call "MCListbox Event - Sort Table.vi"("Clicked Color"=u32 16777216, "Sort Order Boolean Ref"=w431, "MCListBox Ref"=w430) -> ("ItemNames"=w433:string[][])  [unwired: 8 in]
        n208 = Index Array(array=w433, index (col) #1=0 ("disabled index (col)"), index (col) #2=1 ("disabled index (col)")) -> (element #1=w427:string[], element #2=w428:string[])  [unwired: 2 in]
        n209 = Array Size(array=w427) -> (size(s)=w426:i32)
        n210 = case shown="1, Default" w426 {
          tunnel: w428 -> [_ w437]
          tunnel: w427 -> [_ w435]
          frame 0 {
          }
          frame 1, Default {
            n211 = call "String - Array Group By.vi"("Array in"=w435) -> ("GROUP BY (Array in)"=w438:string[])  [unwired: 10 in]
            n212 = call "String - Array Group By.vi"("Array in"=w437) -> ("GROUP BY (Array in)"=w436:string[])  [unwired: 10 in]
            n213 = property on="Search System ID" class="CmbBox (strict)"("Strings[]"=w438) -> ()  [unwired: 2 in, 2 out]
            n214 = property on="Search Equipment ID" class="CmbBox (strict)"("Strings[]"=w436) -> ()  [unwired: 2 in, 2 out]
          }
        }
      }
      event Value Change {
        n215 = event-data() -> ("CtlRef"=w442:refnum<vi>, "NewVal"=w443:T1)  [unwired: 1 in, 4 out]
        n216 = property class="CmbBox (strict)"(reference=w442) -> ("Label.Text"=w441:string)  [unwired: 1 in, 2 out]
        n217 = property class="MCListbox (strict)"(reference=w446) -> ("ItemNames"=w445:string[][])  [unwired: 1 in, 2 out]
        n218 = case shown="\"Search Equipment ID\"" w441 {
          tunnel: [0 ("disabled index (col)") 1 ("disabled index (col)")] -> w440
          frame "Search System ID", Default {
          }
          frame "Search Equipment ID" {
          }
        }
        n219 = Index Array(array=w445, index (col)=w440) -> (element=w444:string[])  [unwired: 1 in]
        n220 = Search 1D Array(1D array=w444, element=w443) -> (index of element=w439:i32)  [unwired: 1 in]
        n221 = case shown="0, Default" w439 {
          tunnel: w439 -> [w447 _]
          frame 0, Default {
            # "Show Searched Row as Top Row"
            # "Leave 5 Rows on top"
            n222 = Subtract(x=w447, y=5) -> (x-y=w449:i32)
            n223 = Greater Or Equal To 0?(x=w449) -> (x >= 0?=w450:bool)
            n224 = Select(t=w449, s=w450, f=0) -> ()  [unwired: 1 out]
            n225 = Bundle("index of element"=w447, 0) -> (w451:cluster{"index of element":i32, i32})  [unwired: 1 in]
            n226 = property on="Multicolumn Listbox" class="MCListbox (strict)"("Val(Sgnl)"=w447, "TopLeft"=w451) -> ()  [unwired: 2 in, 2 out]
          }
          frame -1 {
            # "Combination Not Found"
            n227 = property on="Multicolumn Listbox" class="MCListbox (strict)"("Val(Sgnl)"=-1 ("Value (Signaling)"), "TopLeft"=T5 {"Row"=0, "Column"=0} ("Top Left Visible Cell")) -> ()  [unwired: 2 in, 2 out]
          }
        }
      }
      event "Cal. History": Value Change {
        n228 = event-data() -> ()  [unwired: 1 in, 6 out]
        n229 = property on="Equipment Name" class="Str"() -> ("Text.Text"=w458:string)  [unwired: 2 in, 2 out]
        n230 = property on="Equipment ID" class="Str"() -> ("Text.Text"=w459:string)  [unwired: 2 in, 2 out]
        n231 = call "DB UI - Calibration History.vi"("EquipmentID Description"=w458, "[EquipmentId]"=w459) -> ()  [unwired: 8 in, 2 out]
      }
      event "Current Record": Value Change {
        n232 = event-data() -> ()  [unwired: 1 in, 6 out]
        n233 = local read "Record Count"() -> (w463:i32)
        n234 = In Range and Coerce(upper limit=w463, x="Current Record", lower limit=1) -> (coerced(x)=w464:i32, In Range?=w460:bool)
        n235 = control-ref of="Current Record"() -> (w462:refnum<vi>)
        n236 = case shown="False" w460 {
          tunnel: w468 -> [w471 w472]
          tunnel: w464 -> [w469 w473]
          tunnel: [w471 w472] -> w467
          tunnel: w466 -> [_ _]
          tunnel: "Current Record" -> [_ _]
          tunnel: w462 -> [w470 w474]
          frame False {
            # "To fire an event again so\nthat the calling VIs gets notified\n\nIt may mean that the same record will \nbe fetched again"
            # "Coerce back to Record #"
            n237 = property class="DigNum (strict)"(reference=w470, "Val(Sgnl)"=w469) -> ()  [unwired: 1 in, 2 out]
          }
          frame True {
            # "Valid Record#"
            n238 = property class="DigNum (strict)"(reference=w474, "Value"=w473) -> ()  [unwired: 1 in, 2 out]
          }
        }
      }
      event "Multicolumn Listbox": Value Change {
        # "USER Clicks on MCListbox\nDisable Save, Updates Details Header Cluster"
        n239 = event-data() -> ("Time"=→"MCListBox":u32, "NewVal"=w476:i32)  [unwired: 1 in, 4 out]
        "NewVal" <- w476
        n240 = property on="Save" class="Bool"("DisabledEnum"=T6."Disabled and Grayed Out" ("Disabled")) -> ()  [unwired: 2 in, 2 out]
        n241 = case shown="0, Default" w476 {
          selector: w476 -> [w481 _]
          frame 0, Default {
            n242 = local read "New Record in UI not in DB"() -> (w482:bool)
            n243 = case shown="True" w482 {
              frame False {
                # "Current Record Count is correct"
              }
              frame True {
                # "Current Record Count must -1 since New Record\nno longer available and NOT in DB"
                n244 = local read "Record Count"() -> (w487:i32)
                n245 = local write "New Record in UI not in DB"(FALSE ("New Record in UI not in DB")) -> ()
                n246 = Decrement(x=w487) -> (x-1=w486:i32)
                n247 = local write "Record Count"(w486) -> ()
              }
            }
            n248 = Increment(x=w481) -> (x+1=w480:i32)
            n249 = property on="Cal. History" class="Bool"("DisabledEnum"=T6."Enabled" ("Disabled")) -> ()  [unwired: 2 in, 2 out]
            n250 = property on="Equipment Details Cluster" class="Clust (strict)"() -> (error out=w483:errorcluster, "Controls[]"=w484:refnum<vi>[])  [unwired: 2 in, 1 out]
            n251 = local write "Current Record"(w480) -> ()
            n252 = for {
              tunnel: w484 -> [w503] mode=indexing
              tunnel: w481 -> [w490]
              tunnel: [w496] -> w479
              tunnel: w483 -> [w494]
              n253 = property on="Multicolumn Listbox" class="MCListbox (strict)"() -> ("ColHdrString"=w502:string[], "ItemNames"=w491:string[][])  [unwired: 2 in, 2 out]
              n254 = Index Array(array=w491, index (row)=w490, index (col)=1 ("disabled index (col)")) -> (element=w488:string)
              n255 = Index Array(array=w491, index (row)=w490, index (col)=0 ("disabled index (col)")) -> (element=w492:string)
              n256 = property on="Search System ID" class="CmbBox (strict)"("Value"=w492) -> ()  [unwired: 2 in, 2 out]
              n257 = property on="Search Equipment ID" class="CmbBox (strict)"("Value"=w488) -> ()  [unwired: 2 in, 2 out]
              n258 = property class="Ctl"(reference=w503, error in=w494) -> (reference out=w497:refnum<vi>, error out=w495:errorcluster, "Label.Text"=w501:string)
              n259 = local read "Col Hdrs[] DB Data Type"() -> (w498:string[])
              n260 = Search 1D Array(1D array=w502, element=w501) -> (index of element=w499:i32)  [unwired: 1 in]
              n261 = Greater Or Equal To 0?(x=w499) -> (x >= 0?=w500:bool)
              n262 = case shown="True" w500 {
                tunnel: w491 -> [_ w515]
                tunnel: w490 -> [_ w514]
                tunnel: w499 -> [_ w512]
                tunnel: w498 -> [_ w513]
                tunnel: w497 -> [_ w510]
                tunnel: [w504 w507] -> w496
                tunnel: w495 -> [w504 w506]
                frame False {
                }
                frame True {
                  # "Not used"
                  n263 = Index Array(array=w515, index (row)=w514, index (col)=w512) -> (element=w511:string)
                  n264 = Index Array(array=w513, index=w512) -> ()  [unwired: 1 out]
                  n265 = property class="Ctl"(reference=w510, error in=w506) -> (reference out=w508:refnum<vi>, error out=w505:errorcluster, "ClassName"=w509:string)
                  n266 = case shown="\"AbsTime\"" w509 {
                    tunnel: w511 -> [w518 w530 w536]
                    tunnel: w508 -> [w519 w524 w540]
                    tunnel: [w517 w521 w537] -> w507
                    tunnel: w505 -> [w516 w520 _]
                    frame "False", Default {
                      n267 = property class="Ctl"(reference=w519, error in=w516, "Value"=w518) -> (error out=w517:errorcluster)  [unwired: 1 out]
                    }
                    frame "Boolean" {
                      w525 = refnum<vi> refnum  # Boolean
                      n268 = Equal?(x="1", y=w530) -> (x = y?=w528:bool)
                      n269 = Select(t=TRUE, s=w528, f=FALSE) -> (s? t:f=w522:bool)
                      n270 = To More Specific Class(target class=w525, reference=w524) -> (specific class reference=w523:refnum<vi>)  [unwired: 1 in, 1 out]
                      n271 = property class="Bool"(reference=w523, error in=w520, "Value"=w522) -> (error out=w521:errorcluster)  [unwired: 1 out]
                    }
                    frame "AbsTime" {
                      w539 = refnum<vi> refnum  # AbsTime
                      n272 = call "String - Convert Str (YYYY-mm-dd HHcMMcSS) to TimeStamp.vi"("YYYY-mm-dd HH:MM:SS (String)"=w536) -> ("time stamp"=w531:timestamp)  [unwired: 9 in, 1 out]
                      n273 = To More Specific Class(target class=w539, reference=w540) -> (specific class reference=w538:refnum<vi>)  [unwired: 1 in, 1 out]
                      n274 = Greater?(x=w531, y=timestamp(31593600 s since 1904-01-01)) -> (0:w534:bool)
                      n275 = Select(t=w531, s=w534, f=timestamp(0 s since 1904-01-01) ("time stamp")) -> (s? t:f=w533:timestamp)
                      n276 = property class="AbsTime"(reference=w538, "Value"=w533) -> (error out=w537:errorcluster)  [unwired: 1 in, 1 out]
                    }
                  }
                }
              }
            }
            n277 = local write "Property Node"(w479) -> ()
          }
          frame -1 {
            w541 = ""
            n278 = property on="Search Equipment ID" class="CmbBox (strict)"("Value"=w541) -> ()  [unwired: 2 in, 2 out]
            n279 = property on="Search System ID" class="CmbBox (strict)"("Value"=w541) -> ()  [unwired: 2 in, 2 out]
            n280 = property on="Save" class="Bool"("DisabledEnum"=T6."Disabled and Grayed Out" ("Disabled")) -> ()  [unwired: 2 in, 2 out]
          }
        }
      }
      event "------------------------------------        User Details Header EVENTS     ------------------------------------": Value Change {
        # "DUMMY EVENT"
        n281 = event-data() -> ()  [unwired: 1 in, 6 out]
      }
      event Mouse Down? {
        # "Query for Values of EquipmentTypeId OR SystemId OR PlantId \nto populate their respective ComboBox"
        n282 = event-data() -> ("CtlRef"=w557:refnum<vi>)  [unwired: 1 in, 7 out]
        n283 = property class="CmbBox (strict)"(reference=w557) -> ("Label.Text"=w555:string)  [unwired: 1 in, 2 out]
        n284 = Search 1D Array(1D array=w556, element=w555) -> (index of element=w554:i32)  [unwired: 1 in]
        n285 = Index Array(array=w553, index=w554) -> (element=w543:string)
        n286 = case shown="\"SystemId\"" w543 {
          tunnel: [w572 w573 "SRTRS.Config.Plant" ("DB.Schema.Table 4")] -> w547
          tunnel: ["USE [<DB>]\n\nSELECT [<A>]\nFROM [<Schema>].[<Table>]\n\nWHERE [Inactive] = '0'\nGROUP BY [<A>]\n" "USE [<DB>]\n\nSELECT [<A>]\nFROM [<Schema>].[<Table>]\n\nWHERE [PlantId] = '<B>' AND [Inactive] = '0'\nGROUP BY [<A>]\n" "USE [<DB>]\n\nSELECT [<A>]\nFROM [<Schema>].[<Table>]\n\nWHERE [Inactive] = '0'\nGROUP BY [<A>]\n"] -> w546
          frame "EquipmentTypeId", Default {
            n287 = local read "DB.Schema.Table 2"() -> (w572:string)
          }
          frame "SystemId" {
            n288 = local read "DB.Schema.Table 3"() -> (w573:string)
          }
          frame "PlantId" {
          }
        }
        n289 = call "DB - Split DB.Schema.Table.vi"("DB.Schema.Table"=w547) -> ("DB.Schema.Table"=w563:T11)  [unwired: 10 in]
        n290 = call "DB - Replace DB.Schema.Table.vi"("DB.Schema.Table"=w563, "string in"=w546) -> ("string out"=w552:string)  [unwired: 8 in, 1 out]
        n291 = Search and Replace String(replace all?=TRUE ("replace all? (F)"), input string=w552, search string="<A>", replace string=w543) -> (result string=w551:string)  [unwired: 4 in, 3 out]
        n292 = property on="Plant ID" class="CmbBox (strict)"() -> ("Value"=w544:T1)  [unwired: 2 in, 2 out]
        n293 = Search and Replace String(input string=w551, search string="<B>", replace string=w544) -> (result string=w550:string)  [unwired: 5 in, 3 out]
        n294 = call-poly <vilib>:"DB Tools Execute Query.vi"("SQL query"=w550, "connection reference"=w564) -> ("error out"=w570:errorcluster, "recordset reference"=w569:T12)  [unwired: 6 in]
        n295 = call-poly <vilib>:"DB Tools Fetch Recordset Data.vi"("error in (no error)"=w570, "recordset reference"=w569) -> ("error out"=w565:errorcluster, "recordset data"=w568:variant[][], "recordset reference out"=w566:T12)  [unwired: 3 in]
        n296 = xnode "Database Variant To Data"("database variant"=w568, "type"=string[][] []) -> ("data"=w561:string[][])  [unwired: 1 in, 1 out]
        n297 = call-poly <vilib>:"DB Tools Free Object.vi"("error in (no error)"=w565, "recordset reference"=w566) -> ("error out"=w545:errorcluster)  [unwired: 8 in, 1 out]
        n298 = Index Array(array=w561, index (col)=0 ("disabled index (col)")) -> (element=w559:string[])  [unwired: 1 in]
        n299 = local write "SQL Query"(w550) -> ()
        n300 = local write "DB"(w545) -> ()
        n301 = property class="CmbBox (strict)"(reference=w557, error in=w545, "Strings[]"=w559) -> (error out=w558:errorcluster)  [unwired: 1 out]
        n302 = global write "Global SRTRS.vi" "DB Error"(w545) -> ()
        n303 = local write "Property Node"(w558) -> ()
        n304 = event-data() -> ()  [unwired: 2 in, 1 out]
      }
      event Value Change {
        # "Query for Description of [EquipmentTypeId] OR [SystemId] (no [PlantId])"
        n305 = event-data() -> ("CtlRef"=w654:refnum<vi>)  [unwired: 1 in, 5 out]
        n306 = property class="CmbBox (strict)"(reference=w654) -> ("Label.Text"=w652:string, "Value"=w626:T1)  [unwired: 1 in, 2 out]
        n307 = Search 1D Array(1D array=w653, element=w652) -> (index of element=w651:i32)  [unwired: 1 in]
        n308 = Index Array(array=w650, index=w651) -> (element=w649:string)
        n309 = Format Into String "[Column Name]"(w649) -> (resulting string=w621:string)  [unwired: 3 in, 1 out]
        n310 = case "[Column]" shown="\"SystemId\", Default" w621 {
          tunnel: [w655 w659] -> w631
          tunnel: [w656 w660] -> w625
          tunnel: ["USE [<DB>]\n\nSELECT [Description]\nFROM [<Schema>].[<Table>]\n\nWHERE [<A>] = '<B>' AND [PlantID] = '<C>' AND [Inactive] = '0'\n\n" "USE [<DB>]\n\nSELECT [ShortDescription]\nFROM [<Schema>].[<Table>]\n\nWHERE [<A>] = '<B>' AND [Inactive] = '0'\n\n"] -> w622
          frame "SystemId", Default {
            n311 = control-ref of="System Name"() -> (w656:refnum<vi>)
            n312 = local read "DB.Schema.Table 3"() -> (w655:string)
          }
          frame "EquipmentTypeId" {
            n313 = local read "DB.Schema.Table 2"() -> (w659:string)
            n314 = control-ref of="Equipment Type Name"() -> (w660:refnum<vi>)
          }
        }
        n315 = call "DB - Split DB.Schema.Table.vi"("DB.Schema.Table"=w631) -> ("DB.Schema.Table"=w642:T11)  [unwired: 10 in]
        n316 = call "DB - Replace DB.Schema.Table.vi"("DB.Schema.Table"=w642, "string in"=w622) -> ("string out"=w635:string)  [unwired: 8 in, 1 out]
        n317 = Search and Replace String(replace all?=TRUE ("replace all? (F)"), input string=w635, search string="<A>", replace string=w621) -> (result string=w634:string)  [unwired: 4 in, 3 out]
        n318 = Search and Replace String(input string=w634, search string="<B>", replace string=w626) -> (result string=w629:string)  [unwired: 5 in, 3 out]
        n319 = property on="Plant ID" class="CmbBox (strict)"() -> ("Value"=w623:T1)  [unwired: 2 in, 2 out]
        n320 = Search and Replace String(input string=w629, search string="<C>", replace string=w623) -> (result string=w628:string)  [unwired: 5 in, 3 out]
        n321 = call-poly <vilib>:"DB Tools Execute Query.vi"("SQL query"=w628, "connection reference"=w630) -> ("error out"=w648:errorcluster, "recordset reference"=w647:T12)  [unwired: 6 in]
        n322 = call-poly <vilib>:"DB Tools Fetch Recordset Data.vi"("error in (no error)"=w648, "recordset reference"=w647) -> ("error out"=w643:errorcluster, "recordset data"=w646:variant[][], "recordset reference out"=w644:T12)  [unwired: 3 in]
        n323 = xnode "Database Variant To Data"("database variant"=w646, "type"=string[][] []) -> ("data"=w640:string[][])  [unwired: 1 in, 1 out]
        n324 = call-poly <vilib>:"DB Tools Free Object.vi"("error in (no error)"=w643, "recordset reference"=w644) -> ("error out"=w636:errorcluster)  [unwired: 8 in, 1 out]
        n325 = Index Array(array=w640, index (row)=0 ("disabled index (row)"), index (col)=0 ("disabled index (col)")) -> (element=w638:string)
        n326 = local write "DB"(w636) -> ()
        n327 = local write "SQL Query"(w628) -> ()
        n328 = property class="Str"(reference=w625, error in=w636, "Value"=w638) -> (error out=w637:errorcluster)  [unwired: 1 out]
        n329 = global write "Global SRTRS.vi" "DB Error"(w636) -> ()
        n330 = local write "Property Node"(w637) -> ()
      }
      event "Equipment Details Cluster": Value Change {
        w706 = string[] ["Last Calibration", "Next Calibration"]  # Calibration Fields
        w707 = string[] ["Equipment ID", "Equipment Type", "Plant ID", "Serial Number"]  # Mandatory Fields
        # "Domain ID not used here"
        # "Any Changes in Cluster will fire this event. However we cannot detect which Control in the Cluster has changed. \nEach Control in the Cluster must have their own EVENT Change if we want to process that EVENT individually\nSet Save to Enabled if All mandatory Fields filled"
        n331 = event-data() -> ("Time"=→"User Details":u32)  [unwired: 1 in, 5 out]
        n332 = property on="Domain ID" class="CmbBox (strict)"() -> ("Value"=w714:T1)  [unwired: 2 in, 2 out]
        n333 = property on="Required Calibration" class="Bool (strict)"() -> ("Value"=w708:bool)  [unwired: 2 in, 2 out]
        n334 = Equal?(x=w714, y="Local") -> ()  [unwired: 1 out]
        n335 = property on="Property Node" class="MCListbox (strict)"(reference=w720) -> ("Value"=w719:i32)  [unwired: 1 in, 2 out]
        n336 = control-ref of="Equipment Details Cluster"() -> (w717:refnum<vi>)
        n337 = case shown="True" w708 {
          tunnel: w707 -> [w722 w725]
          tunnel: [w722 w724] -> w705
          tunnel: w706 -> [_ w723]
          frame False {
          }
          frame True {
            n338 = Build Array (concatenate)(w725, w723) -> (w724:string[])
          }
        }
        n339 = property class="Clust (strict)"(reference=w717) -> ("Controls[]"=w716:refnum<vi>[])  [unwired: 1 in, 2 out]
        n340 = Less Than 0?(x=w719) -> (x < 0?=w718:bool)
        n341 = case shown="True" w718 {
          frame False {
          }
          frame True {
            # "No Row Selected, Must be New Record"
            n342 = local read "New Record in UI not in DB"() -> (w766:bool)
            n343 = case shown="False" w766 {
              frame False {
                # "New Record NOT Flagged yet."
                n344 = local read "Record Count"() -> (w768:i32)
                n345 = local write "New Record in UI not in DB"(TRUE ("New Record in UI not in DB")) -> ()
                n346 = Increment(x=w768) -> (x+1=w767:i32)
                n347 = local write "Record Count"(w767) -> ()
                n348 = local write "Current Record"(w767) -> ()
              }
              frame True {
                # "New Record Flagged already\nProbably by NEW Button EVENT"
              }
            }
          }
        }
        n349 = for {
          tunnel: w716 -> [w738] mode=indexing
          tunnel: w705 -> [w736]
          tunnel: [w731] -> w715 mode=indexing
          tunnel: [w732] -> w711 mode=indexing if=w731
          n350 = property class="Ctl"(reference=w738) -> (reference out=w733:refnum<vi>, "Label.Text"=w737:string, "Value"=w734:variant)  [unwired: 1 in, 1 out]
          n351 = Search 1D Array(1D array=w736, element=w737) -> (index of element=w735:i32)  [unwired: 1 in]
          n352 = case shown="0, Default" w735 {
            tunnel: w734 -> [w745 w762 _]
            tunnel: [w741 w758 _] -> w731
            tunnel: w733 -> [w740 w756 _]
            tunnel: [w739 w754 _] -> w732
            frame 0, Default {
              # "Mandatory Fields"
              n353 = Variant To Data(type="", Variant=w745) -> (data=w743:string)  [unwired: 1 in, 1 out]
              n354 = String Length(string=w743) -> (length=w742:i32)
              n355 = case shown="0" w742 {
                tunnel: [TRUE _] -> w741
                tunnel: w740 -> [w749 _]
                tunnel: [w746 _] -> w739
                frame 0 {
                  # "Blank"
                  n356 = property class="Ctl"(reference=w749) -> ("Caption.InterpretAsUnicode"=w748:bool)  [unwired: 1 in, 2 out]
                  n357 = property class="Ctl"(reference=w749) -> ("Caption.Text"=w747:string)  [unwired: 1 in, 2 out]
                  n358 = case shown="False" w748 {
                    tunnel: w747 -> [w752 w753]
                    tunnel: [w751 w753] -> w746
                    frame False {
                      n359 = call "tool_Unicode_Convert ASCII to Unicode (Scalar).vi"("ASCII"=w752) -> ("Unicode"=w751:string)  [unwired: 4 in]
                    }
                    frame True {
                    }
                  }
                }
                frame 1, Default {
                }
              }
            }
            frame 4, 5 {
              # "Last Calibration, Next Calibration"
              n360 = Variant To Data(type=timestamp(0 s since 1904-01-01), Variant=w762) -> (data=w760:timestamp)  [unwired: 1 in, 1 out]
              n361 = Equal?(x=w760, y=timestamp(0 s since 1904-01-01)) -> (x = y?=w758:bool)
              n362 = property class="Ctl"(reference=w756) -> ("Caption.InterpretAsUnicode"=w757:bool)  [unwired: 1 in, 2 out]
              n363 = property class="Ctl"(reference=w756) -> ("Caption.Text"=w755:string)  [unwired: 1 in, 2 out]
              n364 = case shown="False" w757 {
                tunnel: w755 -> [w764 w765]
                tunnel: [w763 w765] -> w754
                frame False {
                  n365 = call "tool_Unicode_Convert ASCII to Unicode (Scalar).vi"("ASCII"=w764) -> ("Unicode"=w763:string)  [unwired: 4 in]
                }
                frame True {
                }
              }
            }
            frame -1 {
            }
          }
        }
        "Controls (Caption) that are blank (Unicode)" <- w711
        n366 = Or Array Elements(Boolean array=w715) -> (logical OR=w709:bool)
        n367 = case shown="True" w709 {
          tunnel: [T6."Enabled" ("Disabled") w728] -> w712
          frame False {
            # "No Blank Mandatory Fields AND\nPassword Match (if Local)"
          }
          frame True {
            # "Blank Mandatory Field exsits OR\nPassword does not match (Local)"
            n368 = Select(t=T6."Disabled and Grayed Out" ("Disabled"), s="Save Enabled depends on \nFilled Mandatory Fields", f=T6."Enabled" ("Disabled")) -> (s? t:f=w728:T6)
          }
        }
        n369 = Not(x=w709) -> (.not. x?=→"All Mandatory Fields Filled":bool)
        n370 = property on="Save" class="Bool"("DisabledEnum"=w712) -> ()  [unwired: 2 in, 2 out]
      }
      event "Equipment Details Cluster.Inactive": Value Change {
        n371 = event-data() -> ("CtlRef"=w770:refnum<vi>, "NewVal"=w771:bool)  [unwired: 1 in, 4 out]
        n372 = case shown="True" w771 {
          tunnel: w770 -> [_ w773]
          frame False {
          }
          frame True {
            n373 = property on="Equipment ID" class="Str"() -> ("Value"=w774:string)  [unwired: 2 in, 2 out]
            n374 = call "Msgbox - Message Handler.vi"("Short Description (When DB Not Available)"="Inactive Equipment", "Description (When DB Not Available)"=" cannot be used after inactive. Do you wish to proceed?", "Pre-Description"=w774, "<.?....> Message Code"="<W 645>") -> ("OK Out"=w772:bool)  [unwired: 5 in, 2 out]
            n375 = property class="Bool (strict)"(reference=w773, "Value"=w772) -> ()  [unwired: 1 in, 2 out]
          }
        }
      }
      event "Equipment Details Cluster.Equipment ID", "Equipment Details Cluster.Manufacturer", "Equipment Details Cluster.Model Number", "Equipment Details Cluster.Serial Number", "Equipment Details Cluster.Last Calibration", "Equipment Details Cluster.Next Calibration", "Equipment Details Cluster.Calibration Period", "Equipment Details Cluster.Notice Period", "Equipment Details Cluster.Registration Date", "Equipment Details Cluster.Remarks": Value Change {
        # "Not in Use"
        # "In this case, only Strings Controls are chosen, so the rest of the cases do not matter."
        # "CAST relevant Controls in Cluster to follow the DB's Length"
        n376 = event-data() -> ("CtlRef"=w782:refnum<vi>)  [unwired: 1 in, 5 out]
        n377 = property on="Property Node" class="MCListbox (strict)"(reference=w779) -> ("ColHdrString"=w781:string[])  [unwired: 1 in, 2 out]
        n378 = property class="Ctl"(reference=w782) -> (reference out=w783:refnum<vi>, "Label.Text"=w778:string, "ClassName"=w789:string, "Value"=w788:variant)  [unwired: 1 in, 1 out]
        n379 = local read "Col Hdrs[] DB Precision"() -> (w786:string[])
        n380 = local read "Col Hdrs[] DB Data Type"() -> (w787:string[])
        n381 = Search 1D Array "Index of Col Hdrs[]"(1D array=w781, element=w778) -> (index of element=w780:i32)  [unwired: 1 in]
        n382 = Index Array(array=w787, index=w780) -> (element=w785:string)
        n383 = Index Array(array=w786, index=w780) -> (element=w784:string)
        n384 = case shown="\"AbsTime\"" w789 {
          tunnel: w788 -> [_ _ _ _ _]
          tunnel: [w799 w826 "" w839 _] -> _
          tunnel: w785 -> [w791 _ _ _ _]
          tunnel: w784 -> [w801 w831 _ _ _]
          tunnel: w783 -> [w794 w836 _ w847 w859]
          tunnel: w778 -> [w792 _ _ _ w854]
          frame "ComboBox", "String" {
            w795 = refnum<vi> refnum  # String
            # "ComboBox may be set to Disallow \"undefined Strings\"\nIf you want to Force to select only listed items in ComboBox"
            n385 = To More Specific Class(target class=w795, reference=w794) -> (specific class reference=w793:refnum<vi>)  [unwired: 1 in, 1 out]
            n386 = case "Special Cases" shown="\"False\", Default" w792 {
              tunnel: w791 -> [w802 _]
              tunnel: [w802 "Numbers & Hyphen"] -> w790
              frame "False", Default {
              }
              frame "Mobile" {
              }
            }
            n387 = property class="Str"(reference=w793) -> (reference out=w800:refnum<vi>, "Value"=w798:string)  [unwired: 1 in, 1 out]
            n388 = Variant To Data(type="", Variant=w798) -> (data=w797:string)  [unwired: 1 in, 1 out]
            n389 = case shown="\"nvarchar\", \"varchar\"" w790 {
              tunnel: w797 -> [_ w807 w810 w817 w823]
              tunnel: w801 -> [_ _ _ w816 w825]
              tunnel: w800 -> [_ w805 _ w814 w821]
              tunnel: [_ w804 w809 w813 w818] -> w799
              frame "False", Default {
                # "unknown"
              }
              frame "Numbers & Hyphen" {
                n390 = Search and Replace String(replace all?=TRUE ("replace all? (F)"), input string=w807, search string="[^0-9-]") -> (result string=w804:string)  [unwired: 5 in, 3 out]
                n391 = property class="Str"(reference=w805, "Value"=w804) -> ()  [unwired: 1 in, 2 out]
              }
              frame "bit" {
                n392 = case shown="\"False\", Default" w810 {
                  tunnel: ["0" "1"] -> w809
                  frame "False", Default {
                  }
                  frame "1", "T", "TRUE", "True" {
                  }
                }
              }
              frame "nvarchar", "varchar" {
                n393 = Decimal String To Number(string=w816) -> (number=w815:i32)  [unwired: 2 in, 1 out]
                n394 = Search/Split String(string=w817, offset (0)=w815) -> (substring before match=w813:string)  [unwired: 1 in, 2 out]
                n395 = property class="Str"(reference=w814, "Value"=w813) -> ()  [unwired: 1 in, 2 out]
              }
              frame "int" {
                n396 = Decimal String To Number(string=w825) -> (number=w824:i32)  [unwired: 2 in, 1 out]
                n397 = Search/Split String(string=w823, offset (0)=w824) -> (substring before match=w822:string)  [unwired: 1 in, 2 out]
                n398 = Decimal String To Number(string=w822) -> (number=w820:i32)  [unwired: 2 in, 1 out]
                n399 = Number To Decimal String(number=w820, width (-)=i16 0) -> (decimal integer string=w818:string)
                n400 = property class="Str"(reference=w821, "Value"=w818) -> ()  [unwired: 1 in, 2 out]
              }
            }
          }
          frame "Digital", "Numeric" {
            w837 = refnum<vi> refnum  # Numeric
            n401 = To More Specific Class(target class=w837, reference=w836) -> (specific class reference=w835:refnum<vi>)  [unwired: 1 in, 1 out]
            n402 = property class="Num"(reference=w835) -> (reference out=w827:refnum<vi>, "Value"=w834:variant)  [unwired: 1 in, 1 out]
            n403 = Variant To Data(type=0, Variant=w834) -> (data=w832:i32)  [unwired: 1 in, 1 out]
            n404 = Format Into String(w832) -> (resulting string=w829:string)  [unwired: 3 in, 1 out]
            n405 = Decimal String To Number(string=w831) -> (number=w830:i32)  [unwired: 2 in, 1 out]
            n406 = Search/Split String(string=w829, offset (0)=w830) -> (substring before match=w826:string)  [unwired: 1 in, 2 out]
            n407 = Decimal String To Number(string=w826) -> (number=w828:i32)  [unwired: 2 in, 1 out]
            n408 = property class="Num"(reference=w827, "Value"=w828) -> ()  [unwired: 1 in, 2 out]
          }
          frame Default {
          }
          frame "Boolean" {
            w846 = refnum<vi> refnum  # Boolean
            n409 = To More Specific Class(target class=w846, reference=w847) -> (specific class reference=w845:refnum<vi>)  [unwired: 1 in, 1 out]
            n410 = property class="Bool"(reference=w845) -> ("Value"=w840:variant)  [unwired: 1 in, 2 out]
            n411 = Variant To Data(type=TRUE, Variant=w840) -> (data=w843:bool)  [unwired: 1 in, 1 out]
            n412 = Select(t="1", s=w843, f="0") -> (s? t:f=w839:string)
          }
          frame "AbsTime" {
            w858 = refnum<vi> refnum  # AbsTime
            n413 = To More Specific Class(target class=w858, reference=w859) -> (specific class reference=w857:refnum<vi>)  [unwired: 1 in, 1 out]
            n414 = property class="AbsTime"(reference=w857) -> (reference out=w848:refnum<vi>, "Value"=w856:variant)  [unwired: 1 in, 1 out]
            n415 = Variant To Data(type=timestamp(0 s since 1904-01-01), Variant=w856) -> (data=w853:timestamp)  [unwired: 1 in, 1 out]
            n416 = case shown="\"Last Calibration\"" w854 {
              tunnel: w853 -> [w871 w878]
              tunnel: [w870 w876] -> w852
              tunnel: ["Invalid Next Calibration Date" "Invalid Last Calibration Date"] -> w851
              tunnel: ["Next calibration cannot be past date." "Last calibration date cannot be future date."] -> w850
              tunnel: ["<E 646>" "<E 643>"] -> w849
              frame "Next Calibration", Default {
                # "Past Date?"
                n417 = Get Date/Time In Seconds() -> (seconds since 1Jan1904=w872:timestamp)
                n418 = Greater?(x=w872, y=w871) -> (0:w870:bool)
              }
              frame "Last Calibration" {
                # "Future Date?"
                n419 = Get Date/Time In Seconds() -> (seconds since 1Jan1904=w877:timestamp)
                n420 = Greater?(x=w878, y=w877) -> (0:w876:bool)
              }
            }
            n421 = case shown="True" w852 {
              tunnel: w851 -> [_ w866]
              tunnel: w850 -> [_ w865]
              tunnel: w849 -> [_ w864]
              tunnel: w848 -> [_ w862]
              frame False {
              }
              frame True {
                # "Date Problems"
                n422 = call "Msgbox - Message Handler.vi"("Short Description (When DB Not Available)"=w866, "Description (When DB Not Available)"=w865, "<.?....> Message Code"=w864) -> ("MHandler Error"=w863:errorcluster)  [unwired: 6 in, 2 out]
                n423 = property class="AbsTime"(reference=w862, "Value"=timestamp(0 s since 1904-01-01)) -> (error out=w860:errorcluster)  [unwired: 1 in, 1 out]
                n424 = local write "MHandler"(w863) -> ()
                n425 = local write "Property Node"(w860) -> ()
              }
            }
          }
        }
      }
      event "------------------------------------------        Unused EVENTS     ----------------------------------------": Value Change {
        # "EVENTS Not used in this VI"
        n426 = event-data() -> ()  [unwired: 1 in, 6 out]
      }
      event "Next Button", "Previous Button", "Last Button", "First Button", "Include Inactive": Value Change {
        # "NOT used in DB UI - Admin User"
        n427 = event-data() -> ("CtlRef"=w879:refnum<vi>)  [unwired: 1 in, 5 out]
        n428 = disable-structure shown="Disabled" {
          disable-tunnel: [w883 _] -> _
          disable-tunnel: w881 -> [w889 _]
          disable-tunnel: w880 -> [w888 _]
          disable-tunnel: w879 -> [w882 _]
          frame Disabled {
            n429 = control-ref of="Include Inactive"() -> (w884:refnum<vi>)
            n430 = local read "New Record in UI not in DB"() -> (w886:bool)
            n431 = Equal?(x=w882, y=w884) -> (x = y?=w883:bool)
            n432 = case shown="True" w886 {
              tunnel: [_ errorcluster {"status"=FALSE, "code"=0, "source"=""} ("error constant")] -> w885
              frame False {
              }
              frame True {
                n433 = local read "Record Count"() -> (w901:i32)
                n434 = local write "New Record in UI not in DB"(FALSE ("New Record in UI not in DB")) -> ()
                n435 = Decrement(x=w901) -> (x-1=w900:i32)
                n436 = local write "Record Count"(w900) -> ()
              }
            }
            n437 = Build Array("First Button", "Previous Button", "Next Button", "Last Button", w883) -> (w894:bool[])
            n438 = Search 1D Array(1D array=w894, element=TRUE) -> (index of element=w887:i32)  [unwired: 1 in]
            n439 = property on="Current Record" class="DigNum (strict)"() -> ("Value"=w898:i32)  [unwired: 2 in, 2 out]
            n440 = case shown="4" w887 {
              tunnel: w898 -> [_ w906 w908 _ w910]
              tunnel: [1 w905 w907 w909 w910] -> w897
              tunnel: w889 -> [_ _ _ _ _]
              tunnel: w888 -> [_ _ _ _ _]
              tunnel: w885 -> [_ _ _ _ _]
              frame 0, Default {
                # "1st Record"
              }
              frame 1 {
                # "Previous"
                n441 = Decrement(x=w906) -> (x-1=w905:i32)
              }
              frame 2 {
                # "Next"
                n442 = Increment(x=w908) -> (x+1=w907:i32)
              }
              frame 3 {
                # "Last Record"
                n443 = local read "Record Count"() -> (w909:i32)
              }
              frame 4 {
                # "Refresh the entireTable because we need to update # of Records also"
                # "Include Invalid"
                n444 = disable-structure shown="Disabled" {
                  frame Disabled {
                    n445 = property on="Property Node" class="CmbBox (strict)"() -> (reference out=w911:refnum<vi>, "Value"=w912:T1)  [unwired: 2 in, 1 out]
                    n446 = property on="Property Node" class="CmbBox (strict)"(reference=w911, "Val(Sgnl)"=w912) -> ()  [unwired: 1 in, 2 out]
                  }
                  frame Enabled {
                  }
                }
              }
            }
            n447 = case shown="0, Default" w887 {
              tunnel: w897 -> [w903 _]
              frame 0, Default {
                # "Update MCListBox"
                n448 = property on="Current Record" class="DigNum (strict)"("Val(Sgnl)"=w903) -> ()  [unwired: 2 in, 2 out]
              }
              frame 4 {
                # "Event already FIRED in Select Table"
              }
            }
            n449 = local write "Changed"(FALSE ("Changed")) -> ()
          }
          frame Enabled {
          }
        }
      }
    }
    "Statemachine" <- w57
  }
  n450 = disable-structure shown="Disabled" {
    frame Disabled {
      w914 = "%Y-%m-%d %H:%M:%S"  # SQL Server datetime
      n451 = Get Date/Time In Seconds() -> (seconds since 1Jan1904=w915:timestamp)
      n452 = Format Date/Time String(time format string (%c)=w914, seconds (now)=w915) -> (date/time string=w913:string)  [unwired: 1 in]
      "datetime string" <- w913
      n453 = Concatenate Strings("INSERT INTO " ("string"), "(TStamp)" ("string"), " values " ("string"), "('" ("string"), w913, "')" ("string")) -> ()  [unwired: 1 in, 1 out]
    }
    frame Enabled {
    }
  }
  n454 = call <vilib>:"DB Tools Close Connection.vi"("error in (no error)"=w7, "connection reference"=w8) -> ("error out"=→"Close":errorcluster)  [unwired: 5 in]
